vi "BIAS.vi"() -> ()   [LabVIEW 2010]
uses:
  <userlib>/bias/subvis/ROI_rect.ctl
  <userlib>/bias/subvis/Imaging_State.ctl
  <userlib>/bias/subvis/Frame_Controls.ctl
  <vilib>/Utility/error.llb/DialogType.ctl
  <userlib>/bias/classes/CameraBase/CameraBase.lvclass
  <vilib>/event_ctls.llb/lveventtype.ctl
  <userlib>/bias/subvis/zlock/ZLock.lvclass
  <userlib>/bias/subvis/ExposureSettings.ctl
  <vilib>/addons/h5labview2/file/H5Fmode.ctl
  <vilib>/addons/h5labview2/base/hid_t.ctl
  <vilib>/addons/h5labview2/attrib/H5Aread.llb/H5Aread.xnode
  <vilib>/addons/h5labview2/dataset/H5Dread.llb/H5Dread.xnode
  <vilib>/addons/h5labview2/attrib/H5Awrite.llb/H5Awrite.xnode
  <vilib>/Utility/file.llb/Read From Spreadsheet File (DBL).vi
  <vilib>/addons/h5labview2/base/lib_path.vi
  <vilib>/addons/h5labview2/base/H5Equery.vi
  <vilib>/Analysis/NI_AALPro.lvlib
  <vilib>/addons/zeromq/zeromq.lvlib
  <vilib>/addons/h5labview2/file/H5F.lvlib
  <vilib>/addons/h5labview2/group/H5G.lvlib
  <vilib>/addons/h5labview2/attrib/H5A.lvlib
panel:
  in  "files":T1 caption="Files"
  in  "stop":bool
  in  "fit_buttons":cluster{"selection":bool, "stored":bool} caption="Fit"
  in  "tools_zoom":T2 caption="Zoom tools"
  in  "tools_view":cluster{"sel":bool, "in":bool, "out":bool} caption="View tools"
  in  "capture":T3 caption="Capture"
  out "stop_time":dbl=11.582550000000003
  out "busy":bool caption="Busy"
  out "recent_error":bool caption="Error"
  out "remote":bool caption="Remote"
  out "acquiring":bool caption="Acquiring"
  out "img_OD":T4(plugin-control)
  out "n_atoms":dbl caption="Atom number:" format="%_4e"
  out "image_raw":sgl[][](array[numeric])
  in  "tabs":T5(tab)
  in  "store_settings":bool
  in  "binning":cluster{"x":u8, "y":u8}={"x"=1, "y"=1}
  in  "newinst":bool
  in  "effective_pixel":dbl caption="effective pixel size"
  in  "rotation":u16(ring) items=["Do not rotate", "Rotate 90°", "Rotate 180°", "Rotate -90°"]
  out "cam_params":cluster{"String":string, "value":variant}[](array[cluster])=[{"String"="TriggerSource", "value"=variant(string "Freerun")}, {"String"="Timeout", "value"=variant(u32 23583)}, {"String"="ShiftPixelBits", "value"=variant(bool FALSE)}, {"String"="PixelFormat", "value"=variant(string "Mono14")}] caption="Camera Parameters"
  in  "rois":T7(array[cluster])=[{"get"=FALSE, "set"=FALSE, "rect"={"left"=0, "top"=0, "right"=0, "bottom"=0}, "color"=16777224}, {"get"=FALSE, "set"=FALSE, "rect"={"left"=0, "top"=0, "right"=0, "bottom"=0}, "color"=6618880}, {"get"=FALSE, "set"=FALSE, "rect"={"left"=0, "top"=0, "right"=0, "bottom"=0}, "color"=16776960}, {"get"=FALSE, "set"=FALSE, "rect"={"left"=0, "top"=0, "right"=0, "bottom"=0}, "color"=4849919}]
  in  "camera name":string
  out "camera model":string="GX1920 (02-2410B), serial 0xF3101FDAB"
  in  "exposure":sgl=100.0 caption="exposure (ms)"
  out "location":string caption="camera location"
  out "roi_sensor":T6={"left"=0, "top"=0, "right"=1936, "bottom"=1456} caption="camera size"
  out "roi_capture":T6={"left"=686, "top"=399, "right"=1281, "bottom"=1004}
  out "keep":u8
  in  "pedestal":u16=100 caption="Camera pedestal value"
  in  "comp_Isat":bool=TRUE caption="compute?"
  in  "Isat":dbl=4300.0
  in  "Icutoff":dbl=500.0 caption="Intensity threshold"
  in  "xsection":dbl=2.9049e-13 caption="Transition Cross-section"
  out "working dir":path
  out "current file":string
  in  "comp_list":i32(listbox) caption="Computed Frames"
  in  "raw_ctrls":T8={"col_scheme"=0, "val_min"=100.0, "val_max"=16384.0, "automax"=FALSE} {"col_scheme" items=["Grayscale", "Rainbow", "Temperature", "-", "AlpineColors", "Amherst", "Aquamarine", "ArmyColors", "AtlanticColors", "AuroraColors", "AvocadoColors", "BeachColors", "BlueGreenYellow", "BrassTones", "BrightBands", "BrownCyanTones", "CandyColors", "CherryTones", "CMYKColors", "CoffeeTones", "DarkBands", "DarkRainbow", "DarkTerrain", "DeepSeaColors", "Default", "FallColors", "FruitPunchColors", "FuchsiaTones", "GrayTones", "GrayYellowTones", "GreenBrownTerrain", "GreenPinkTones", "IslandColors", "LabVIEW", "LakeColors", "LightTemperatureMap", "LightTerrain", "MintColors", "NeonColors", "NIST", "Pastel", "PearlColors", "PigeonTones", "PlumColors", "Rainbow", "RedBlueTones", "RedGreenSplit", "RoseColors", "RustTones", "SandyTerrain", "SiennaTones", "SolarColors", "SouthwestColors", "StarryNightColors", "SunsetColors", "TemperatureMap", "ThermometerColors", "ValentineTones", "WatermelonColors"]; "val_max" format="%_4g"; "val_min" format="%_4g"}
  in  "comp_ctrls":T8={"col_scheme"=39, "val_min"=0.0, "val_max"=3.0, "automax"=FALSE} {"col_scheme" items=["Grayscale", "Rainbow", "Temperature", "-", "AlpineColors", "Amherst", "Aquamarine", "ArmyColors", "AtlanticColors", "AuroraColors", "AvocadoColors", "BeachColors", "BlueGreenYellow", "BrassTones", "BrightBands", "BrownCyanTones", "CandyColors", "CherryTones", "CMYKColors", "CoffeeTones", "DarkBands", "DarkRainbow", "DarkTerrain", "DeepSeaColors", "Default", "FallColors", "FruitPunchColors", "FuchsiaTones", "GrayTones", "GrayYellowTones", "GreenBrownTerrain", "GreenPinkTones", "IslandColors", "LabVIEW", "LakeColors", "LightTemperatureMap", "LightTerrain", "MintColors", "NeonColors", "NIST", "Pastel", "PearlColors", "PigeonTones", "PlumColors", "Rainbow", "RedBlueTones", "RedGreenSplit", "RoseColors", "RustTones", "SandyTerrain", "SiennaTones", "SolarColors", "SouthwestColors", "StarryNightColors", "SunsetColors", "TemperatureMap", "ThermometerColors", "ValentineTones", "WatermelonColors"]; "val_max" format="%_4g"; "val_min" format="%_4g"}
  in  "raw_list":i32(listbox)=-1 caption="Raw Frames"
  in  "alpha":dbl=1.0 caption="Alpha"
  in  "hold_frames":bool caption="Hold last flat/dark frames"
  in  "histograms":bool caption="histogram"
  in  "Save OD":bool=TRUE
  in  "fit_function":enum16{"Gaussian", "ThomasFermi"}(ring)
  in  "fit clip":dbl=5.0 caption="OD clip" min=1.0
  out "fit_current":bool caption="Current"
  out "fit_number":dbl caption="Fitted atom number:"
  in  "bin_size":i32=5 caption="rebin size" min=1
  out "fit_params":T9(array[cluster])=[{"param"="Fit_residuals", "uncert"=0.0, "uncert 2"=0.0}, {"param"="Fit_rebin", "uncert"=0.0, "uncert 2"=0.0}, {"param"="Gaussian_X0", "uncert"=0.12302468141779599, "uncert 2"=0.0}, {"param"="Gaussian_Y0", "uncert"=0.17648801424407168, "uncert 2"=0.0}, {"param"="Gaussian_XW", "uncert"=0.11674772619735485, "uncert 2"=0.0}, {"param"="Gaussian_YW", "uncert"=0.16283739371170114, "uncert 2"=0.0}, {"param"="Gaussian_Amp", "uncert"=0.008479207725537119, "uncert 2"=0.0}, {"param"="Gaussian_Offset", "uncert"=0.003580147540181461, "uncert 2"=0.0}, {"param"="Gaussian_Nint", "uncert"=1132011.7271960815, "uncert 2"=0.0}] caption="Fit Results" {"uncert 2" format="%#_4g"; "uncert" format="%#_4g"}
  in  "auto fit":bool caption="Auto fit"
  out "data points:":u32=7656 caption="Npoints"
  out "Y-lineout":dbl[][](graph)
  out "X-lineout":dbl[][](graph)
  in  "fit_roi":T10={"get"=FALSE, "set"=FALSE, "rect"={"left"=792, "top"=473, "right"=1233, "bottom"=911}, "color"=16711680} caption="Fitting region"
  out "recent":string[](array[string]) caption="recent log messages"
  out "state":T11 caption="system state"
  in  "last error":T12={"status"=FALSE, "code"=42, "description"="", "time"=timestamp(3029490000.67111 s since 1904-01-01)} caption="most recent error:" {"time" format="%<%H:%M:%S %d/%m/%y>T"}
  out "sequencer":T13(array[cluster])
  out "comp_data":T14(array[cluster])
  out "roi_current":T6
  out "image_data":u16[][][](array[numeric])
  out "frame":i32=-1 caption="display_frame"
  out "fit attribs":variant[](array[variant])
  out "BLACS port":u16
  in  "calc timeout":u32=10000
  out "image_size":i32[](array[numeric])
  out "attribs":variant[](array[variant])=[variant(i32 864), variant(i32 519), variant(i32 1176), variant(i32 878), variant(i64 0), variant(string "Freerun"), variant(u32 1), variant(u32 1), variant(i64 864), variant(i64 519), variant(i64 312), variant(i64 359), variant(dbl 100000.00149011612)]
  out "raw histograms":T15(array[cluster])
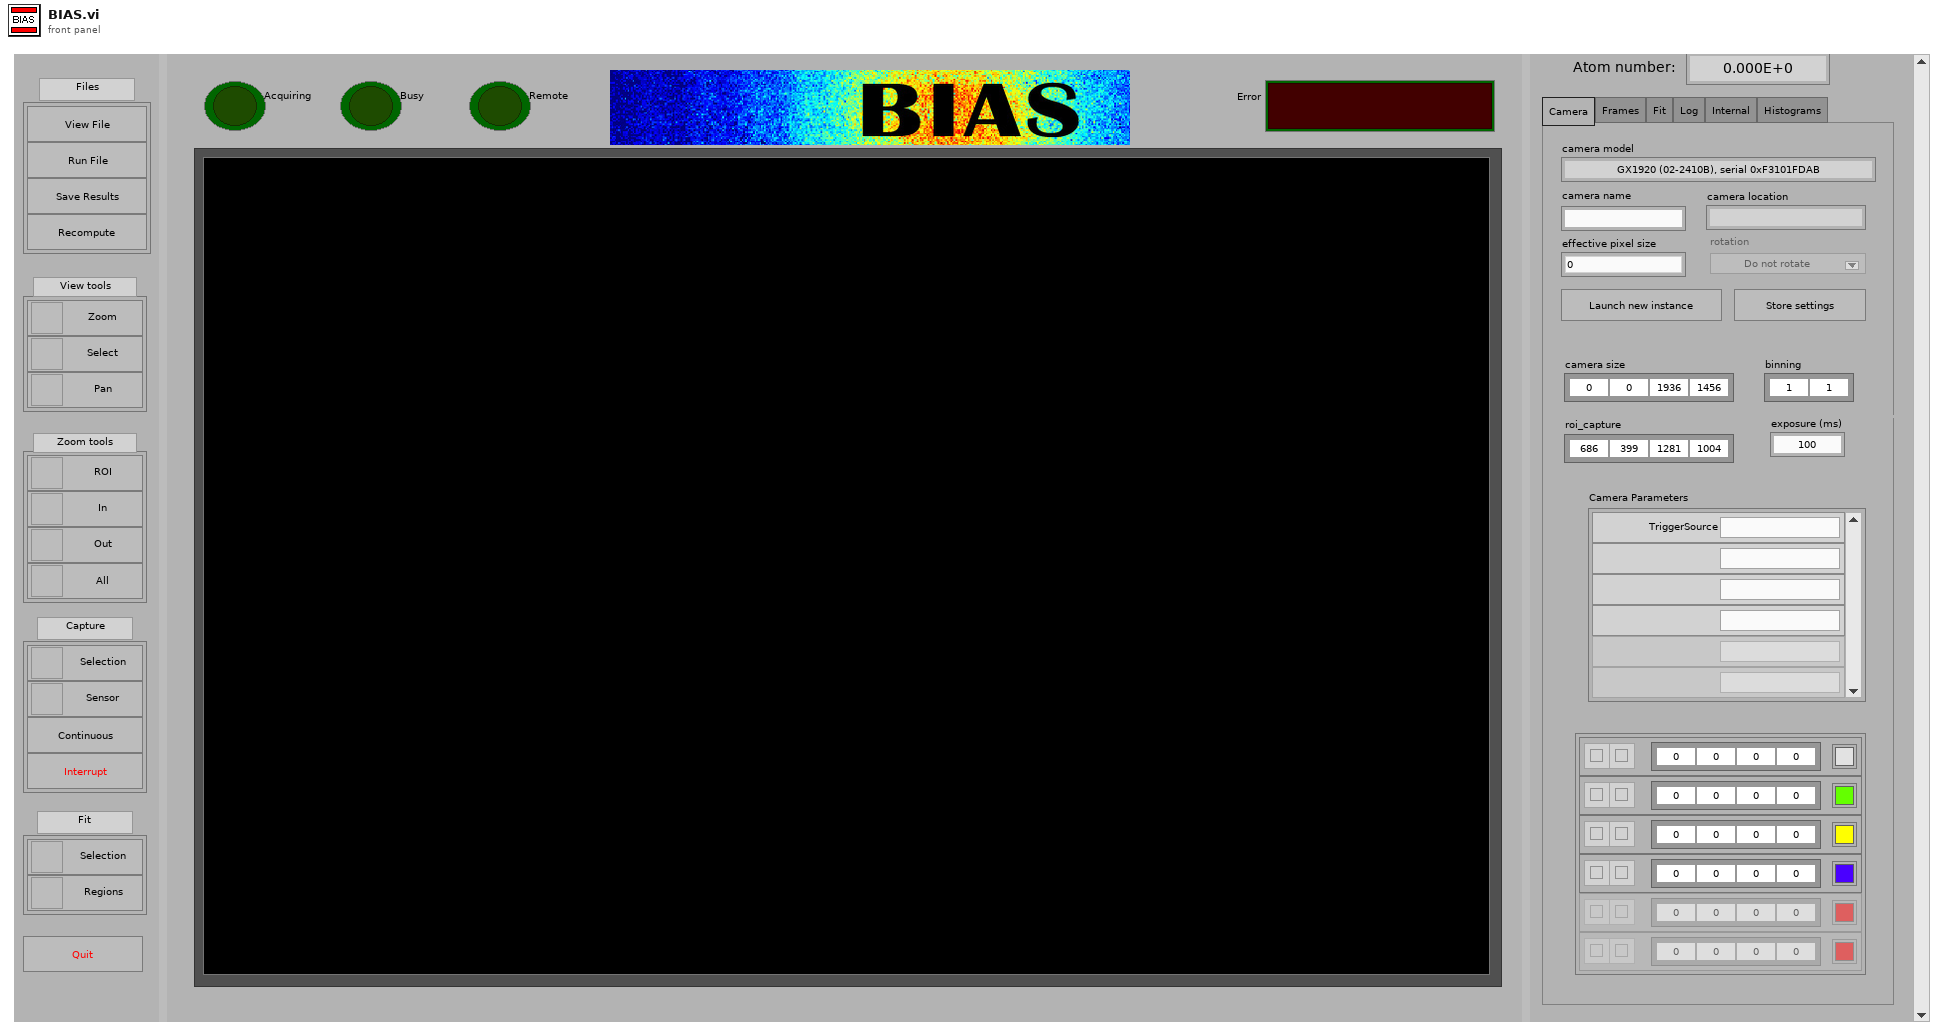
[diagram p1: front panel]
types:
  T1 = cluster{"open_file 2":bool, "open_file":bool, "save_file":bool, "open_file 3":bool}
  T2 = cluster{"sel":bool, "in":bool, "out":bool, "all":bool}
  T3 = cluster{"roi":bool, "chip":bool, "continuous":bool, "abort":bool}
  T4 = typedef "IMAQ Image.ctl" = refnum<image>
  T5 = enum32{"Camera", "Frames", "Fit", "Log", "Internal", "Histograms"}
  T6 = typedef "ROI_rect.ctl" = cluster{"left":i32, "top":i32, "right":i32, "bottom":i32}
  T7 = cluster{"get":bool, "set":bool, "rect":T6, "color":u32}[]
  T8 = typedef "Frame_Controls.ctl" = cluster{"col_scheme":u16, "val_min":sgl, "val_max":sgl, "automax":bool}
  T9 = cluster{"param":string, "uncert":dbl, "uncert 2":dbl}[]
  T10 = cluster{"get":bool, "set":bool, "rect":T6, "color":u32}
  T11 = typedef "Imaging_State.ctl" = enum16{"<NULL>", "Init", "Read File", "Save File", "Idle", "Compute", "Redraw", "Draw Overlays", "Software trigger", "Acquire", "Fit", "Clear", "Quit"}
  T12 = cluster{"status":bool, "code":i32, "description":string, "time":timestamp}
  T13 = cluster{"name":string, "shots":string[], "ids":i32[]}[]
  T14 = cluster{"sequence":string, "name":string, "data":sgl[][], "params":variant[]}[]
  T15 = cluster{"XY Graph":cluster{"X Values":dbl[], "Histogram: h(x)":i32[]}}[]
  T16 = typedef "DialogType.ctl" = u16
  T17 = typedef "pointer.ctl" = u64
  T18 = typedef "ExposureSettings.ctl" = cluster{"exposure":dbl, "external":bool, "roi":T6, "frames":i32, "binning":cluster{"x":u8, "y":u8}}
  T19 = cluster{"Icutoff":dbl, "Isat":dbl, "sigma":dbl, "pixel_size":dbl}
  T20 = typedef "H5F.lvlib/H5Fmode.ctl" = enum16{"read-only", "read-write", "overwrite", "create new", "open or create"}
  T21 = enum8{"Enabled", "Disabled", "Disabled and Grayed Out"}
  T22 = typedef "Image Type" = u32
  T23 = cluster{"sensor_width":u16, "sensor_width":u16, "sensor_width":u16, "sensor_height":u16}
  T24 = cluster{"sequence":string, "name":string, "data":sgl[][], "params":variant[]}
  T25 = cluster{"X Values":dbl[], "Histogram: h(x)":i32[]}
  T26 = cluster{"Histogram Graph":cluster{"X Values":dbl[], "Histogram: h(x)":i32[]}}
  T27 = typedef "hid_t.ctl" = i32
  T28 = cluster{"name":string, "shots":string[], i32[]}[]
  T29 = cluster{"Name":string, "Name":string, "data":sgl[][], "params":variant[]}[]
  T30 = enum32{"Invalid", "Standard", "Closed", "Hidden", "Minimized", "Maximized"}
  T31 = typedef "lveventtype.ctl" = enum32{"Null", "Timeout", "App Instance Close", "App Instance Close?", "Autoscale Range Change", "Cell Edit", "Cell Edit?", "Cursor Grab", "Cursor Grab?", "Cursor Move", "Cursor Release", "Data Change", "Direction Change", "Display State Change", "Drag Ended", "Drag Enter", "Drag Leave", "Drag Over", "Drag Source Update", "Drag Starting", "Drag Starting?", "Drop", "Exec State Change", "Key Down", "Key Down?", "Key Repeat", "Key Repeat?", "Key Up", "Listbox Double Click", "Menu Activation?", "Menu Selection (App)", "Menu Selection? (App)", "Menu Selection (User)", "Mouse Down", "Mouse Down?", "Mouse Enter", "Mouse Leave", "Mouse Move", "Mouse Up", "NI Security User Change (App)", "Pane Size", "Panel Close", "Panel Close?", "Panel Resize", "Plot Attribute Change", "Scale Range Change", "Shortcut Menu Activation?", "Shortcut Menu Selection (App)", "Shortcut Menu Selection? (App)", "Shortcut Menu Selection (User)", "Tree Double Click", "Tree Drag", "Tree Drag?", "Tree Drop", "Tree Drop?", "Tree Item Close", "Tree Item Close?", "Tree Item Open", "Tree Item Open?", "Value Change"}
  T32 = cluster{"Global Rectangle":i32[], "Contours":cluster{"Contour Type":u32, "ROI Type":u32, "Points":i32[]}[]}
  T33 = typedef "ROI Descriptor" = cluster{"Global Rectangle":i32[], "Contours":cluster{"ID":enum32{"External", "Internal"}, "Type":u32, "Coordinates":i32[]}[]}
  T34 = cluster{"Contour Type":u32, "ROI Type":u32, "Points":i32[]}[]
  T35 = cluster{"FinalVal[0]":bool, "FinalVal[1]":bool, "FinalVal[2]":bool}
  T36 = cluster{"all rows[0]":dbl, "all rows[1]":dbl, "all rows[2]":dbl}
  T37 = cluster{"Value":u8, "Value":u8, "Value":u8, "Value":u8}
  T38 = enum16{"Standard", "Buffered", "CRLF", "Immediate"}
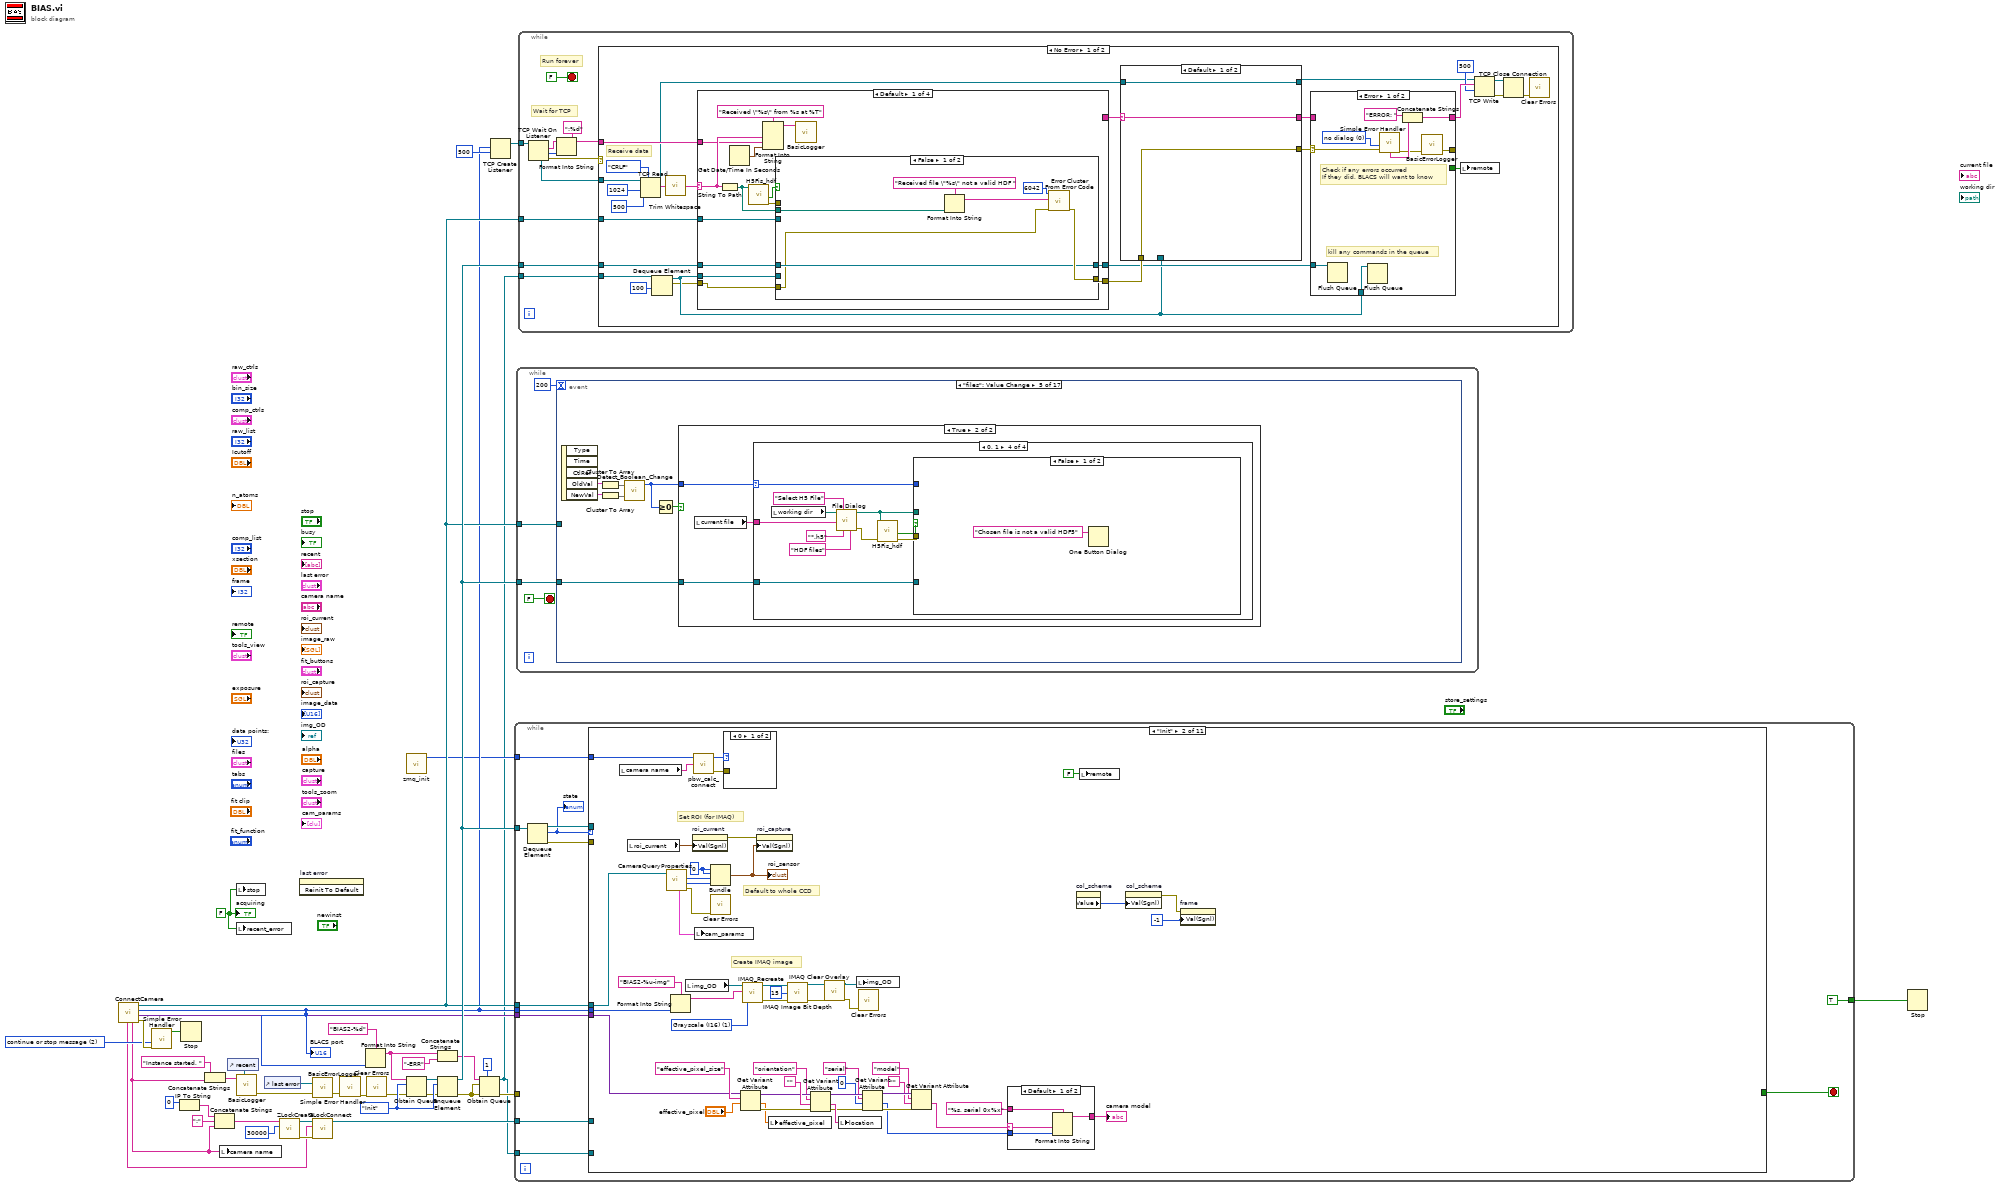
[diagram p0: block diagram]
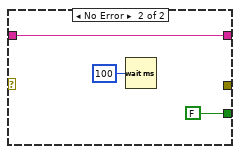
[diagram p2: hidden frame]
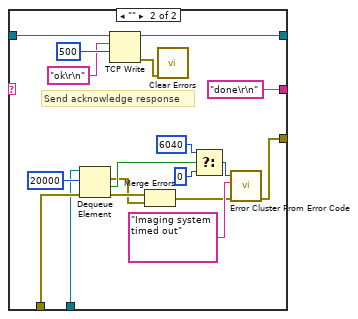
[diagram p3: hidden frame]
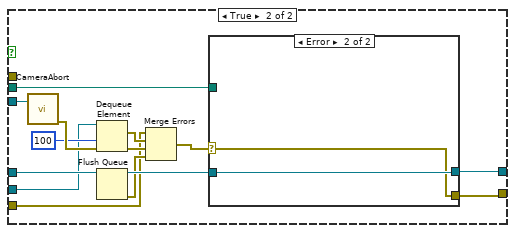
[diagram p4: hidden frame]
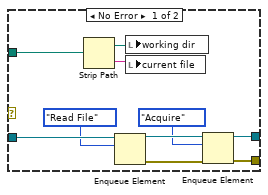
[diagram p5: hidden frame]
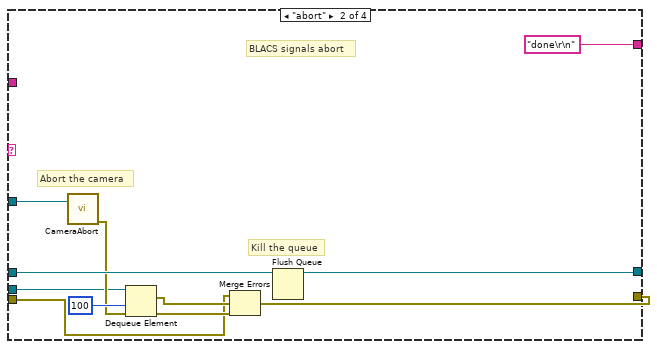
[diagram p6: hidden frame]
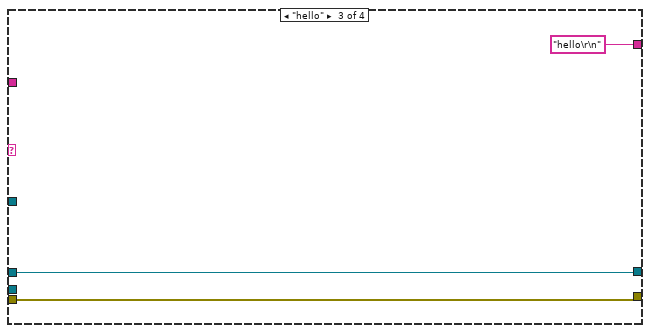
[diagram p7: hidden frame]
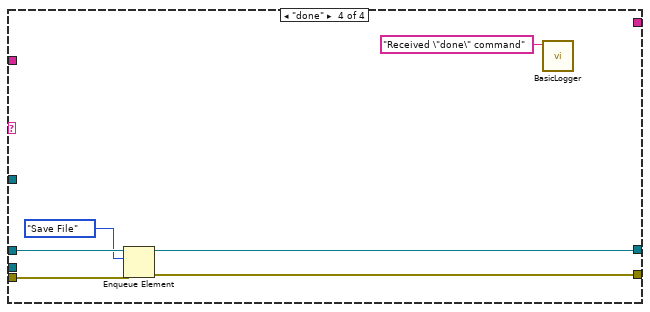
[diagram p8: hidden frame]
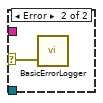
[diagram p9: hidden frame]
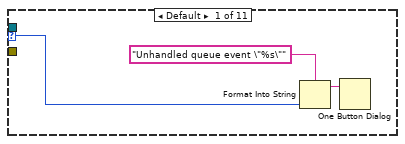
[diagram p10: hidden frame]
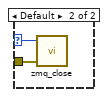
[diagram p11: hidden frame]
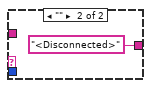
[diagram p12: hidden frame]
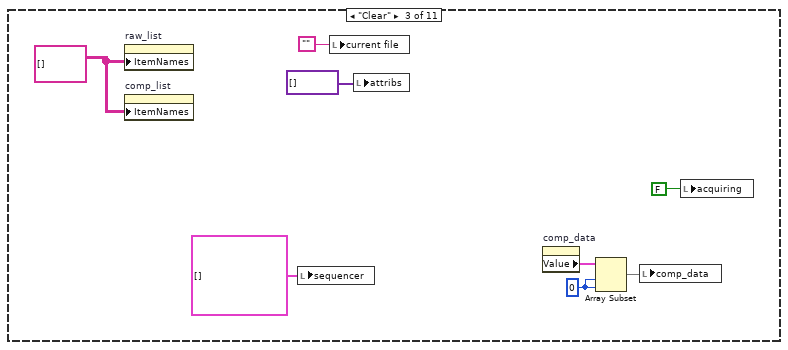
[diagram p13: hidden frame]
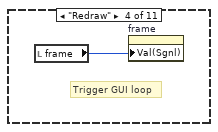
[diagram p14: hidden frame]
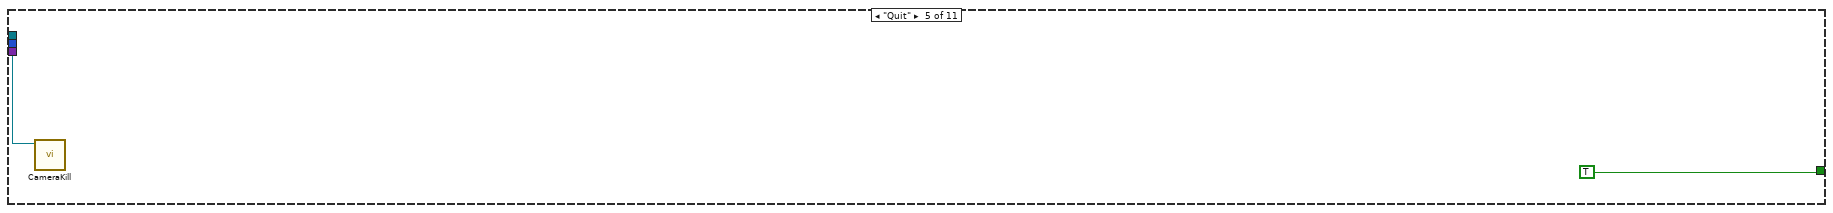
[diagram p15: hidden frame]
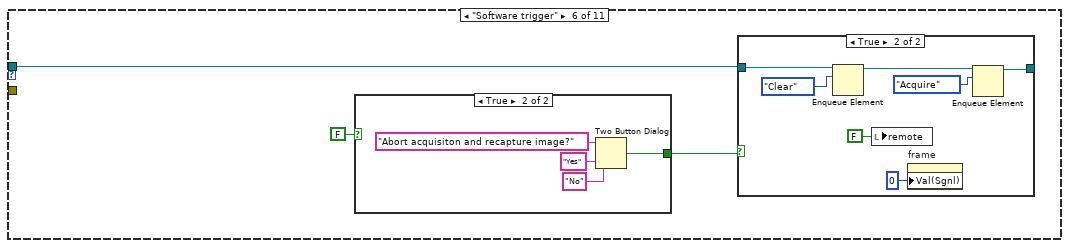
[diagram p16: hidden frame]
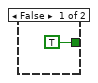
[diagram p18: hidden frame]
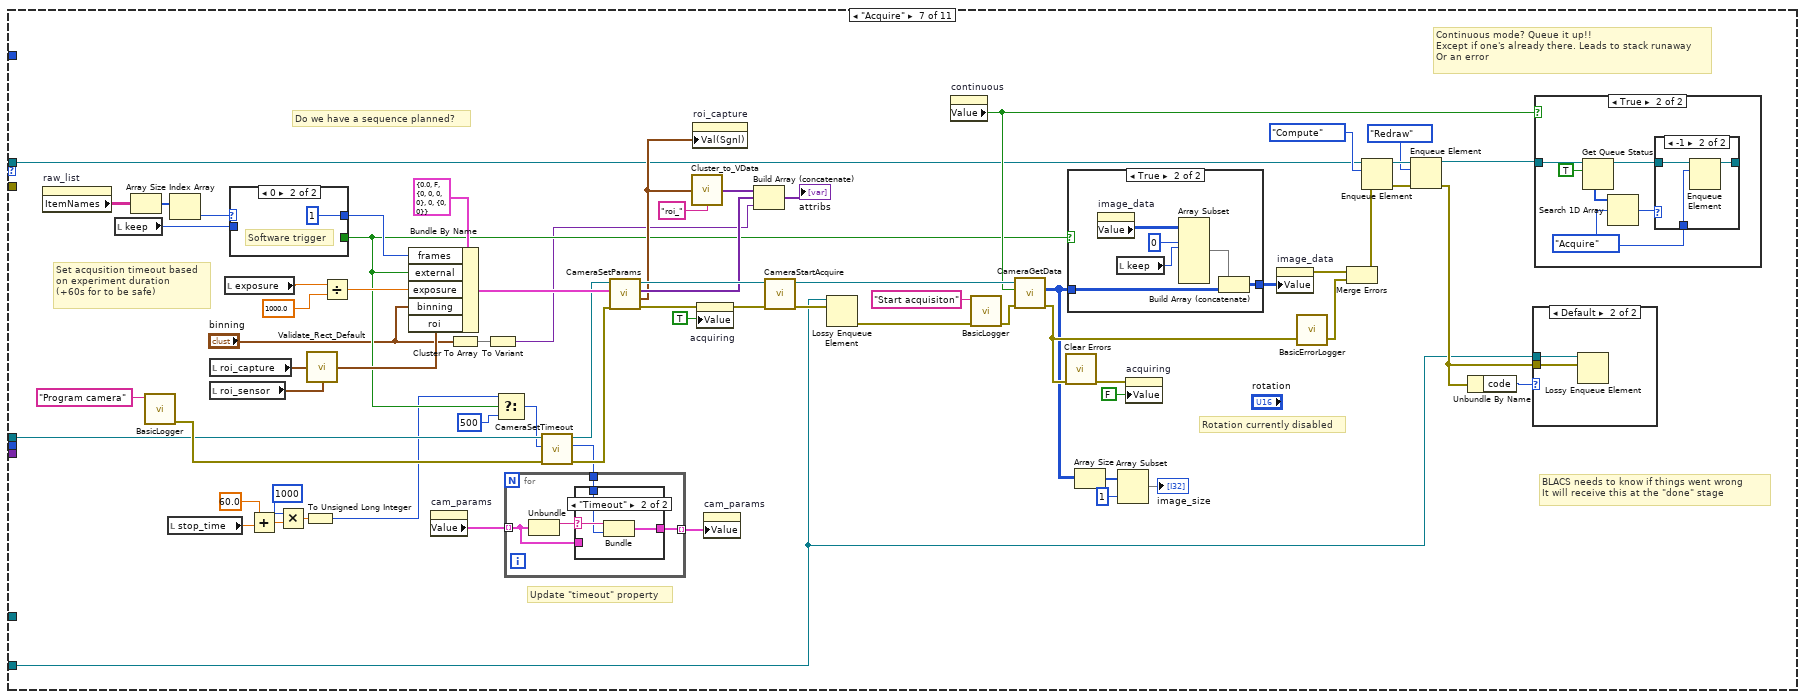
[diagram p19: hidden frame]
diagram:
  w20 = T16 2 items=["no dialog", "OK message", "continue or stop message", "OK message + warnings", "continue/stop + warnings"] ("type of dialog (OK msg:1)")
  w26 = FALSE ("acquiring")
  w40 = Imaging_State."Init" ("Imaging_State")
  n1 = call <userlib>:"ConnectCamera.vi"() -> ("error out"=w22:errorcluster, "params"=w10:variant, "port"=w23:u16, "camera"=w24:refnum<class "CameraBase.lvclass">, "camera name"=w9:string, "zlock"=w11:string)  [unwired: 3 in, 1 out]
  "BLACS port" <- w23
  n2 = call <vilib>:"Simple Error Handler.vi"("type of dialog (OK msg:1)"=w20, "error in (no error)"=w22) -> ("error?"=w21:bool)  [unwired: 3 in, 4 out]
  n3 = IP To String(2:u32 0 ("net address")) -> (0:w15:string)  [unwired: 1 in]
  n4 = Stop(stop? (T)=w21) -> ()
  n5 = Concatenate Strings("Instance started, " ("string"), w9) -> (w27:string)
  n6 = Concatenate Strings(w15, ":" ("string"), w9) -> (w16:string)
  n7 = local write "camera name"(w9) -> ()
  n8 = control-ref of="recent"() -> (w29:refnum<vi>)
  n9 = local write "stop"(w26) -> ()
  n10 = local write "recent_error"(w26) -> ()
  n11 = call <userlib>:"BasicLogger.vi"("indicator"=w29, "text"=w27) -> ("error out"=w30:errorcluster)  [unwired: 5 in, 1 out]
  n12 = control-ref of="last error"() -> (w34:refnum<vi>)
  n13 = call <userlib>:"ZLockCreate.vi"("timeout (500ms)"=30000, "app name"=w16) -> ("error out"=w18:errorcluster, "ZLock out"=w19:refnum<class "ZLock.lvclass">)  [unwired: 4 in]
  n14 = invoke on="last error" class="Clust (strict)" method="Reinit To Default"() -> ()  [unwired: 3 in, 3 out]
  n15 = call <userlib>:"BasicErrorLogger.vi"("error in"=w30, "indicator"=w34) -> ("error out"=w33:errorcluster)  [unwired: 1 out]
  n16 = call-dynamic "ZLockConnect.vi"("error in (no error)"=w18, "host"=w11, "ZLock in"=w19) -> ("ZLock out"=w17:refnum<class "ZLock.lvclass">)  [unwired: 7 in, 1 out]
  n17 = call <vilib>:"Simple Error Handler.vi"("error in (no error)"=w33) -> ("error out"=w32:errorcluster)  [unwired: 4 in, 4 out]
  n18 = Format Into String(format string="BIAS2-%d" ("name (unnamed)"), w23) -> (resulting string=w7:string)  [unwired: 2 in, 1 out]
  n19 = call <vilib>:"Clear Errors.vi"("error in (no error)"=w32) -> ("error out"=w31:errorcluster)  [unwired: 6 in]
  n20 = call <vilib>:"zmq_init.vi"() -> ("context"=w12:T17)  [unwired: 4 in, 1 out]
  n21 = Obtain Queue(name (unnamed)=w7, element data type=w40, error in (no error)=w31) -> (queue out=w41:refnum<queue>, error out=w39:errorcluster)  [unwired: 2 in, 1 out]
  n22 = Concatenate Strings(w7, "-ERR" ("name (unnamed)")) -> (w5:string)
  n23 = Enqueue Element(queue=w41, element=w40, error in (no error)=w39) -> (queue out=w36:refnum<queue>, error out=w4:errorcluster)  [unwired: 1 in, 1 out]
  n24 = Obtain Queue(max queue size (-1, unlimited)=1, name (unnamed)=w5, element data type=w4, error in (no error)=w4) -> (queue out=w1:refnum<queue>, error out=w8:errorcluster)  [unwired: 1 in, 1 out]
  n25 = TCP Create Listener(9:500 ("timeout ms (25000)"), 10:w23) -> (3:w35:refnum<k5>)  [unwired: 3 in, 2 out]
  n26 = while {
    tunnel: [TRUE] -> w38
    tunnel: w24 -> [w49]
    tunnel: w36 -> [w44]
    tunnel: w12 -> [w48]
    tunnel: w17 -> [w47]
    tunnel: w23 -> [w46]
    tunnel: w10 -> [w43]
    tunnel: w8 -> [_]
    tunnel: w1 -> [w42]
    stop <- w50 stop-if-true
    n27 = Dequeue Element(queue=w44) -> (queue out=w53:refnum<queue>, element=w45:T11, error out=w52:errorcluster)  [unwired: 2 in, 1 out]
    "state" <- w45
    n28 = case shown="\"Init\"" w45 {
      selector: w45 -> [w55 _ _ _ _ _ _ _ _ _ _]
      tunnel: w53 -> [_ _ _ _ _ w126 w145 w251 _ w439 w673]
      tunnel: w52 -> [_ _ _ _ _ _ _ _ _ _ _]
      tunnel: [_ _ _ _ TRUE _ _ _ _ _ _] -> w50
      tunnel: w49 -> [_ w89 _ _ w123 _ w179 _ _ _ _]
      tunnel: w48 -> [_ w82 _ _ _ _ _ w245 w346 _ _]
      tunnel: w47 -> [_ _ _ _ _ _ _ _ _ w434 w674]
      tunnel: w46 -> [_ w79 _ _ _ _ _ _ _ _ _]
      tunnel: w43 -> [_ w63 _ _ _ _ _ _ _ _ _]
      tunnel: w42 -> [_ _ _ _ _ _ w141 _ _ w433 w672]
      frame Default {
        n29 = Format Into String(format string="Unhandled queue event \"%s\"", w55) -> (resulting string=w54:string)  [unwired: 2 in, 1 out]
        n30 = One Button Dialog(message=w54) -> ()  [unwired: 1 in, 1 out]
      }
      frame "Init" {
        w88 = u16 0 ("sensor_width")
        w105 = T22 1 items=["Grayscale (U8)", "Grayscale (I16)", "Grayscale (SGL)", "Complex (CSG)", "RGB (U32)", "HSL (U32)", "RGB (U64)", "Grayscale (U16)"] ("type")
        # "Create IMAQ image"
        # "Default to whole CCD"
        # "Set ROI (for IMAQ)"
        n31 = local read "camera name"() -> (w80:string)
        n32 = local read "roi_current"() -> (w100:T6)
        n33 = call-dynamic "CameraQueryProperties.vi"("CameraBase in"=w89) -> ("error out"=w90:errorcluster, "sensor_height"=w99:u16, "sensor_width"=w98:u16, "cam_params"=w97:cluster{"String":string, "value":variant}[])  [unwired: 6 in, 1 out]
        n34 = Format Into String(format string="BIAS2-%u-img", w79) -> (resulting string=w83:string)  [unwired: 2 in, 1 out]
        n35 = local read "img_OD"() -> (w106:T4)
        n36 = property on="roi_current" class="Clust (strict)"("Val(Sgnl)"=w100) -> (error out=w101:errorcluster)  [unwired: 2 in, 1 out]
        n37 = call <userlib>:"pbw_calc_connect.vi"("identity"=w80, "ctx in"=w82) -> ("error out"=w81:errorcluster, "socket out"=w57:T17)  [unwired: 2 in]
        n38 = local write "cam_params"(w97) -> ()
        n39 = Bundle("sensor_width"=w88, "sensor_width"=w88, "sensor_width"=w98, "sensor_height"=w99) -> (w85:T23)  [unwired: 1 in]
        "roi_sensor" <- w85
        n40 = call <vilib>:"Clear Errors.vi"("error in (no error)"=w90) -> ()  [unwired: 6 in, 1 out]
        n41 = case shown="0" w57 {
          selector: w57 -> [_ w107]
          tunnel: w81 -> [_ w108]
          frame 0 {
          }
          frame Default {
            n42 = call <vilib>:"zmq_close.vi"("error in"=w108, "socket in"=w107) -> ()  [unwired: 3 in, 1 out]
          }
        }
        n43 = Get Variant Attribute(Variant=w63, name="effective_pixel_size", default value (empty Variant)="effective_pixel") -> (duplicate Variant=w72:variant, value=w65:dbl, error out=w75:errorcluster)  [unwired: 1 in, 1 out]
        n44 = call <userlib>:"IMAQ_Recreate.vi"("type"=w105, "name"=w83, "image in"=w106) -> ("error out"=w102:errorcluster, "image out"=w104:T4)  [unwired: 3 in]
        n45 = property on="roi_capture" class="Clust (strict)"(error in=w101, "Val(Sgnl)"=w85) -> ()  [unwired: 1 in, 2 out]
        n46 = local write "effective_pixel"(w65) -> ()
        n47 = call "IMAQ Image Bit Depth"("Image"=w104, "Bit Depth (0)"=u32 15, "error in (no error)"=w102) -> ("Image Out"=w95:T4, "error out"=w96:errorcluster)  [unwired: 10 in, 1 out]
        n48 = Get Variant Attribute(Variant=w72, name="orientation", default value (empty Variant)="", error in=w75) -> (duplicate Variant=w73:variant, value=w77:string, error out=w76:errorcluster)  [unwired: 1 out]
        n49 = call "IMAQ Clear Overlay"("error in (no error)"=w96, "Image"=w95) -> ("error out"=w93:errorcluster, "Image Out"=w94:T4)  [unwired: 8 in]
        n50 = local write "location"(w77) -> ()
        n51 = local write "img_OD"(w94) -> ()
        n52 = call <vilib>:"Clear Errors.vi"("error in (no error)"=w93) -> ()  [unwired: 6 in, 1 out]
        n53 = Get Variant Attribute(Variant=w73, name="serial", default value (empty Variant)=u64 0, error in=w76) -> (duplicate Variant=w70:variant, value=w68:u64, error out=w71:errorcluster)  [unwired: 1 out]
        n54 = Get Variant Attribute(Variant=w70, name="model", default value (empty Variant)="", error in=w71) -> (value=w69:string)  [unwired: 3 out]
        n55 = case shown="Default" w69 {
          selector: w69 -> [w110 _]
          tunnel: [w112 "<Disconnected>"] -> w59
          tunnel: w68 -> [w111 _]
          tunnel: "%s, serial 0x%x" ("format string") -> [w109 _]
          frame Default {
            n56 = Format Into String(format string=w109, w110, w111) -> (resulting string=w112:string)  [unwired: 2 in, 1 out]
          }
          frame "" {
          }
        }
        "camera model" <- w59
        n57 = property on="col_scheme" class="Ring (strict)"() -> ("Value"=w91:u16)  [unwired: 2 in, 2 out]
        n58 = local write "remote"(FALSE ("remote")) -> ()
        n59 = property on="col_scheme" class="Ring (strict)"("Val(Sgnl)"=w91) -> (error out=w86:errorcluster)  [unwired: 2 in, 1 out]
        n60 = property on="frame" class="DigNum (strict)"(error in=w86, "Val(Sgnl)"=-1 ("display_frame")) -> ()  [unwired: 1 in, 2 out]
      }
      frame "Clear" {
        w116 = 0 ("index")
        w119 = string[][] [] ("sequence")
        n61 = property on="raw_list" class="MCListbox (strict)"("ItemNames"=w119) -> ()  [unwired: 2 in, 2 out]
        n62 = property on="comp_list" class="MCListbox (strict)"("ItemNames"=w119) -> ()  [unwired: 2 in, 2 out]
        n63 = local write "sequencer"(T13 [] ("sequencer")) -> ()
        n64 = local write "current file"("") -> ()
        n65 = local write "attribs"(variant[] []) -> ()
        n66 = property on="comp_data" class="Arr (strict)"() -> ("Value"=w114:T14)  [unwired: 2 in, 2 out]
        n67 = Array Subset(array=w114, index=w116, length=w116) -> (w117:T14)
        n68 = local write "comp_data"(w117) -> ()
        n69 = local write "acquiring"(FALSE ("pending")) -> ()
      }
      frame "Redraw" {
        # "Trigger GUI loop"
        n70 = local read "frame"() -> (w122:i32)
        n71 = property on="frame" class="DigNum (strict)"("Val(Sgnl)"=w122) -> ()  [unwired: 2 in, 2 out]
      }
      frame "Quit" {
        n72 = call-dynamic "CameraKill.vi"("CameraBase in"=w123) -> ()  [unwired: 9 in, 2 out]
      }
      frame "Software trigger" {
        n73 = case shown="True" FALSE {
          tunnel: [TRUE ("T button?") w137] -> w127
          frame False {
          }
          frame True {
            n74 = Two Button Dialog(message="Abort acquisiton and recapture image?", 1:"No" ("F button name (\"Cancel\")"), 2:"Yes" ("T button name (\"OK\")")) -> (T button?=w137:bool)
          }
        }
        n75 = case shown="True" w127 {
          tunnel: [w128 w134] -> _
          tunnel: w126 -> [w128 w133]
          frame False {
          }
          frame True {
            n76 = Enqueue Element(queue=w133, element=Imaging_State."Clear") -> (queue out=w132:refnum<queue>)  [unwired: 2 in, 2 out]
            n77 = local write "remote"(FALSE ("remote")) -> ()
            n78 = property on="frame" class="DigNum (strict)"("Val(Sgnl)"=0 ("Value (Signaling)")) -> ()  [unwired: 2 in, 2 out]
            n79 = Enqueue Element(queue=w132, element=Imaging_State."Acquire") -> (queue out=w134:refnum<queue>)  [unwired: 2 in, 2 out]
          }
        }
      }
      frame "Acquire" {
        # "Update \"timeout\" property"
        # "Rotation currently disabled"
        # "Set acqusition timeout based\non experiment duration\n(+60s for to be safe)"
        # "BLACS needs to know if things went wrong\nIt will receive this at the \"done\" stage"
        # "Continuous mode? Queue it up!!\nExcept if one's already there. Leads to stack runaway\nOr an error"
        # "Do we have a sequence planned?"
        n80 = property on="raw_list" class="MCListbox (strict)"() -> ("ItemNames"=w190:string[][])  [unwired: 2 in, 2 out]
        n81 = local read "keep"() -> (w183:u8)
        n82 = Array Size(array=w190) -> (size(s)=w189:i32[])
        n83 = call <userlib>:"BasicLogger.vi"("text"="Program camera") -> ("error out"=w180:errorcluster)  [unwired: 6 in, 1 out]
        n84 = local read "stop_time"() -> (w174:dbl)
        n85 = Index Array(array=w189) -> (element=w188:i32)  [unwired: 1 in]
        n86 = local read "roi_capture"() -> (w204:T6)
        n87 = local read "roi_sensor"() -> (w199:T6)
        n88 = local read "exposure"() -> (w208:sgl)
        n89 = case shown="0" w188 {
          selector: w188 -> [w237 _]
          tunnel: [w238 1] -> w165
          tunnel: [TRUE ("external") _] -> w156
          tunnel: w183 -> [w236 _]
          frame Default {
            n90 = Subtract(x=w237, y=w236) -> (x-y=w238:i32)
          }
          frame 0 {
            # "Software trigger"
          }
        }
        n91 = Add(x=60.0, y=w174) -> (x+y=w175:dbl)
        n92 = Multiply(x=u32 1000 ("col"), y=w175) -> (x*y=w182:dbl)
        n93 = To Unsigned Long Integer(number=w182) -> (unsigned 32bit integer=w155:u32)
        n94 = call <userlib>:"Validate_Rect_Default.vi"("rect"=w204, "default"=w199) -> ("out"=w169:T6)
        n95 = Divide(x=w208, y=sgl 1000.0) -> (x/y=w203:sgl)
        n96 = Bundle By Name(cluster=T18 {"exposure"=0.0, "external"=FALSE, "roi"={"left"=0, "top"=0, "right"=0, "bottom"=0}, "frames"=0, "binning"={"x"=0, "y"=0}} ("settings"), "frames"=w165, "external"=w156, "exposure"=w203, "binning"="binning", "roi"=w169) -> (w202:T18)
        n97 = property on="cam_params" class="Arr (strict)"() -> ("Value"=w164:cluster{"String":string, "value":variant}[])  [unwired: 2 in, 2 out]
        n98 = Cluster To Array(cluster="binning") -> (array=w146:u8[])
        n99 = To Variant(anything=w146) -> (Variant=w147:variant)
        n100 = Select(t=w155, s=w156, f=u32 500) -> (s? t:f=w154:u32)
        n101 = call-dynamic "CameraSetTimeout.vi"("error in (no error)"=w180, "Timeout"=w154, "CameraBase in"=w179) -> ("error out"=w178:errorcluster, "Timeout set"=w176:u32, "CameraBase out"=w177:refnum<class "CameraBase.lvclass">)  [unwired: 6 in]
        n102 = for {
          tunnel: w164 -> [w216] mode=indexing
          tunnel: w176 -> [w217]
          tunnel: [w219] -> w163 mode=indexing
          n103 = Unbundle(w216) -> ("String"=w218:string)  [unwired: 1 out]
          n104 = case shown="\"Timeout\"" w218 {
            selector: w218 -> [_ w222]
            tunnel: [w220 w223] -> w219
            tunnel: w217 -> [_ w221]
            tunnel: w216 -> [w220 _]
            frame Default {
            }
            frame "Timeout" {
              n105 = Bundle(w222, "Timeout set"=w221) -> (w223:cluster{string, "Timeout set":u32})  [unwired: 1 in]
            }
          }
        }
        n106 = call-dynamic "CameraSetParams.vi"("error in (no error)"=w178, "settings"=w202, "CameraBase in"=w177) -> ("error out"=w195:errorcluster, "roi_out"=w171:T6, "attributes"=w187:variant[], "CameraBase out"=w194:refnum<class "CameraBase.lvclass">)  [unwired: 5 in]
        n107 = call <userlib>:"Cluster_to_VData.vi"("cluster"=w171, "prefix"="roi_") -> ("vdata"=w186:variant[])
        n108 = property on="roi_capture" class="Clust (strict)"("Val(Sgnl)"=w171) -> ()  [unwired: 2 in, 2 out]
        n109 = property on="acquiring" class="Bool (strict)"(error in=w195, "Value"=TRUE ("acquiring")) -> (error out=w192:errorcluster)  [unwired: 1 in, 1 out]
        n110 = property on="cam_params" class="Arr (strict)"("Value"=w163) -> ()  [unwired: 2 in, 2 out]
        n111 = Build Array (concatenate)(w186, w187, w147) -> (→"attribs":variant[])
        n112 = call-dynamic "CameraStartAcquire.vi"("error in (no error)"=w192, "CameraBase in"=w194) -> ("error out"=w143:errorcluster, "CameraBase out"=w193:refnum<class "CameraBase.lvclass">)  [unwired: 8 in]
        n113 = Lossy Enqueue Element(queue=w141, element=w143) -> (error out=w144:errorcluster)  [unwired: 1 in, 3 out]
        n114 = property on="continuous" class="Bool (strict)"() -> ("Value"=w168:bool)  [unwired: 2 in, 2 out]
        n115 = call <userlib>:"BasicLogger.vi"("error in"=w144, "text"="Start acquisiton") -> ("error out"=w191:errorcluster)  [unwired: 5 in, 1 out]
        n116 = call-dynamic "CameraGetData.vi"("error in (no error)"=w191, "keep open?"=w168, "CameraBase in"=w193) -> ("error out"=w206:errorcluster, "image_data"=w152:u16[][][])  [unwired: 6 in, 1 out]
        n117 = call <vilib>:"Clear Errors.vi"("error in (no error)"=w206) -> ("error out"=w196:errorcluster)  [unwired: 6 in]
        n118 = case shown="True" w156 {
          tunnel: [w209 w212] -> w172
          tunnel: w152 -> [w209 w210]
          frame False {
          }
          frame True {
            n119 = property on="image_data" class="Arr (strict)"() -> ("Value"=w211:u16[][][])  [unwired: 2 in, 2 out]
            n120 = local read "keep"() -> (w214:u8)
            n121 = Array Subset(array=w211, index (dim 0)=0 ("index"), length (dim 0)=w214) -> (w213:u16[][][])  [unwired: 4 in]
            n122 = Build Array (concatenate)(w213, w210) -> (w212:u16[][][])
          }
        }
        n123 = Array Size(array=w152) -> (size(s)=w151:i32[])
        n124 = Array Subset(array=w151, index=1) -> (→"image_size":i32[])  [unwired: 1 in]
        n125 = property on="acquiring" class="Bool (strict)"(error in=w196, "Value"=FALSE ("acquiring")) -> ()  [unwired: 1 in, 2 out]
        n126 = property on="image_data" class="Arr (strict)"("Value"=w172) -> (error out=w167:errorcluster)  [unwired: 2 in, 1 out]
        n127 = call <userlib>:"BasicErrorLogger.vi"("error in"=w206) -> ("error out"=w166:errorcluster)  [unwired: 1 in, 1 out]
        n128 = Merge Errors(w167, w166) -> (w159:errorcluster)
        n129 = Enqueue Element(queue=w145, element=Imaging_State."Compute", error in (no error)=w159) -> (queue out=w162:refnum<queue>, error out=w158:errorcluster)  [unwired: 1 in, 1 out]
        n130 = Enqueue Element(queue=w162, element=Imaging_State."Redraw", error in (no error)=w158) -> (queue out=w142:refnum<queue>, error out=w157:errorcluster)  [unwired: 1 in, 1 out]
        n131 = Unbundle By Name(w157) -> ("code"=w184:i32)
        n132 = case shown="Default" w184 {
          tunnel: w157 -> [_ w225]
          tunnel: w141 -> [_ w224]
          frame 0, 5024 {
            # "Fine or Abort"
          }
          frame Default {
            n133 = Lossy Enqueue Element(queue=w224, element=w225) -> ()  [unwired: 1 in, 4 out]
          }
        }
        n134 = case shown="True" w168 {
          tunnel: w142 -> [_ w231]
          frame False {
          }
          frame True {
            w226 = Imaging_State."Acquire" ("element")
            n135 = Get Queue Status(queue=w231, return elements? (F)=TRUE) -> (queue out=w227:refnum<queue>, elements=w229:T11[])  [unwired: 1 in, 6 out]
            n136 = Search 1D Array(1D array=w229, element=w226) -> (index of element=w228:i32)  [unwired: 1 in]
            n137 = case shown="-1" w228 {
              tunnel: [w232 w235] -> _
              tunnel: w227 -> [w232 w234]
              tunnel: w226 -> [_ w233]
              frame Default {
              }
              frame -1 {
                n138 = Enqueue Element(queue=w234, element=w233) -> (queue out=w235:refnum<queue>)  [unwired: 2 in, 2 out]
              }
            }
          }
        }
      }
      frame "Compute" {
        # ">> num frames >>"
        # "Ensure the fit happens before saving if auto fit enabled."
        n139 = property on="comp_data" class="Arr (strict)" props=["Value"]() -> ()  [unwired: 2 in, 3 out]
        n140 = property on="sequencer" class="Arr (strict)"() -> ("Value"=w246:T13)  [unwired: 2 in, 2 out]
        n141 = property on="raw_list" class="MCListbox (strict)"() -> ("ItemNames"=w254:string[][])  [unwired: 2 in, 2 out]
        n142 = local read "camera name"() -> (w241:string)
        n143 = for {
          N -> [w281]
          tunnel: w246 -> [w285] mode=indexing
          tunnel: [w291] -> w249
          tunnel: w254 -> [w288]
          tunnel: [errorcluster {"status"=FALSE, "code"=0, "source"=""} ("error in (no error)")] -> w250
          tunnel: [w281] -> w252
          tunnel: w245 -> [w280]
          shift-right: [w278] -> w243
          shift-left: T14 [] -> [w279]
          tunnel: w241 -> [w277]
          # ">> sequence >>"
          # "Try to find frames"
          n144 = Unbundle(w285) -> ("name"=w292:string)  [unwired: 2 out]
          n145 = call <userlib>:"Keep_Find.vi"("x"="atoms" ("name"), "sequence"=w285) -> ("index"=w283:i32)  [unwired: 1 in]
          n146 = call <userlib>:"Keep_Find.vi"("x"="flat" ("name"), "rawlist"=w288, "sequence"=w285) -> ("index"=w287:i32)
          n147 = call <userlib>:"Keep_Find.vi"("x"="dark" ("name"), "rawlist"=w288, "sequence"=w285) -> ("index"=w286:i32)
          n148 = Greater Or Equal To 0?(x=w283) -> (x >= 0?=w295:bool)
          n149 = Greater Or Equal To 0?(x=w287) -> (x >= 0?=w294:bool)
          n150 = Compound Arithmetic op=AND(w295, w294) -> (w293:bool)
          n151 = case shown="True" w293 {
            tunnel: w283 -> [_ w334]
            tunnel: w287 -> [_ w332]
            tunnel: w286 -> [_ w333]
            tunnel: w292 -> [_ w331]
            tunnel: [_ w321] -> w291
            tunnel: w280 -> [_ w303]
            tunnel: w279 -> [w296 w298]
            tunnel: [w296 w299] -> w278
            tunnel: w277 -> [_ w297]
            frame False {
            }
            frame True {
              w310 = 1 ("dimension size")
              n152 = property on="image_data" class="Arr (strict)"() -> ("Value"=w314:u16[][][])  [unwired: 2 in, 2 out]
              n153 = local read "effective_pixel"() -> (w301:dbl)
              n154 = Index Array(array=w314, index (dim 0) #1=w334, index (dim 0) #2=w332, index (dim 0) #3=w333) -> (element #1=w304:u16[][], element #2=w305:u16[][], element #3=w307:u16[][])  [unwired: 6 in]
              n155 = local read "xsection"() -> (w318:dbl)
              n156 = Select(t="Isat", s="comp_Isat", f=0.0) -> (s? t:f=w319:dbl)
              n157 = local read "Icutoff"() -> (w320:dbl)
              n158 = Empty Array?(array=w307) -> (empty?=w309:bool)
              n159 = Initialize Array("pedestal", w310, w310) -> (w308:u16[][])
              n160 = Bundle By Name(cluster=T19 {"Icutoff"=0.0, "Isat"=0.0, "sigma"=0.0, "pixel_size"=0.0} ("params"), "Icutoff"=w320, "Isat"=w319, "sigma"=w318, "pixel_size"=w301) -> (w312:T19)
              n161 = Select(t=w308, s=w309, f=w307) -> (s? t:f=w306:u16[][])
              n162 = call <userlib>:"Compute_OD.vi"("dark"=w306, "flat"=w305, "atoms"=w304, "ctx in"=w303, "params"=w312, "identity"=w297, "timeout"="calc timeout") -> ("error out"=w317:errorcluster, "alpha"=w323:dbl, "N"=w321:dbl, "OD"=w322:sgl[][])
              n163 = call <userlib>:"BasicErrorLogger.vi"("error in"=w317) -> ("error out"=w329:errorcluster)  [unwired: 1 in, 1 out]
              n164 = call <vilib>:"Clear Errors.vi"("error in (no error)"=w329) -> ()  [unwired: 6 in, 1 out]
              n165 = local write "alpha"(w323) -> ()
              n166 = call <userlib>:"Set Data Name__ogtk.vi"("Data Name"="atom_number", "Data"=w321) -> ("Renamed Data"=w325:variant)  [unwired: 8 in, 1 out]
              n167 = property class="Clust (strict)"() -> ("Value"=w328:T24)  [unwired: 2 in, 2 out]
              n168 = Build Array(w325) -> (w326:variant[])
              n169 = Bundle(cluster=w328, "sequence"=w331, "name"="OD", "data"=w322, "params"=w326) -> (w300:T24)
              n170 = Build Array (concatenate)(w298, w300) -> (w299:T14)
            }
          }
        }
        "comp_data" <- w243
        n171 = case shown="Default" w252 {
          tunnel: w250 -> [_ w257]
          frame Default {
            n172 = local read "frame"() -> (w256:i32)
            n173 = property on="frame" class="DigNum (strict)"("Val(Sgnl)"=w256) -> ()  [unwired: 2 in, 2 out]
          }
          frame 1.. {
            n174 = property on="comp_list" class="MCListbox (strict)"(error in=w257, "Val(Sgnl)"=0 ("Value (Signaling)")) -> ()  [unwired: 1 in, 2 out]
          }
        }
        n175 = Greater Than 0?(x=w249) -> (x > 0?=w247:bool)
        n176 = for {
          tunnel: w243 -> [w276] mode=indexing
          tunnel: [w275] -> w255 mode=indexing
          n177 = Unbundle(w276) -> ("sequence"=w274:string, "name"=w273:string)  [unwired: 2 out]
          n178 = Build Array(w274, w273) -> (w275:string[])
        }
        n179 = call <userlib>:"GrayOut.vi"("enabled?"=w247) -> ("state"=w248:T21)
        n180 = case shown="True" "histograms" {
          frame False {
          }
          frame True {
            # "Raw image histograms (very slow)"
            n181 = property on="image_data" class="Arr (strict)"() -> ("Value"=w259:u16[][][])  [unwired: 2 in, 2 out]
            n182 = for {
              tunnel: w259 -> [w267] mode=indexing
              tunnel: [w263] -> w260 mode=indexing
              n183 = Array Size(array=w267) -> (size(s)=w269:i32[])
              n184 = Multiply Array Elements(1:w269) -> (0:w268:i32)
              n185 = Reshape Array(w267, w268) -> (w266:u16[])
              n186 = call <vilib>:"General Histogram.vi"("X"=w266, "max"=16384.0, "min"=0.0, "# bins"=400 ("intervals")) -> ("Histogram Graph"=w264:T25)  [unwired: 7 in, 4 out]
              n187 = Bundle("Histogram Graph"=w264) -> (w263:T26)  [unwired: 1 in]
            }
            "raw histograms" <- w260
          }
        }
        n188 = property on="n_atoms" class="DigNum (strict)"("Value"=w249, "DisabledEnum"=w248) -> ()  [unwired: 2 in, 2 out]
        n189 = case shown="True" "auto fit" {
          tunnel: w251 -> [_ w272]
          tunnel: w250 -> [_ w270]
          frame False {
          }
          frame True {
            n190 = Enqueue Element At Opposite End(queue=w272, element=Imaging_State."Fit", error in (no error)=w270) -> ()  [unwired: 1 in, 3 out]
          }
        }
        n191 = property on="comp_list" class="MCListbox (strict)"("ItemNames"=w255) -> ()  [unwired: 2 in, 2 out]
      }
      frame "Fit" {
        n192 = local read "fit_roi"() -> (w369:T10)
        n193 = property on="comp_data" class="Arr (strict)"() -> ("Value"=w348:T14)  [unwired: 2 in, 2 out]
        n194 = local read "frame"() -> (w358:i32)
        n195 = local read "binning"() -> (w335:cluster{"x":u8, "y":u8})
        n196 = property on="image_data" class="Arr (strict)"() -> ("Value"=w349:u16[][][])  [unwired: 2 in, 2 out]
        n197 = local read "roi_capture"() -> (w365:T6)
        n198 = Unbundle By Name(w369) -> ("rect"=w351:T6)
        n199 = Max & Min(x=w358, y=0) -> (max(x,y)=w356:i32)  [unwired: 1 out]
        n200 = Unbundle(w335) -> ("x"=w338:u8, "y"=w339:u8)
        n201 = call <userlib>:"Validate_Rect_Default.vi"("rect"=w351, "default"=w365) -> ("out"=w350:T6)
        n202 = Negate(x=w365) -> (-x=w364:T6)
        n203 = Empty Array?(array=w348) -> (empty?=w362:bool)
        n204 = Bundle("x"=w338, "y"=w339, "x"=w338, "y"=w339) -> (w337:cluster{"x":u8, "y":u8, "x":u8, "y":u8})  [unwired: 1 in]
        n205 = Index Array(array=w348) -> (element=w367:T24)  [unwired: 1 in]
        n206 = Index Array(array=w349, index (dim 0)=w356) -> (element=w359:u16[][])  [unwired: 2 in]
        n207 = Unbundle By Name(w367) -> ("data"=w361:sgl[][])
        n208 = call <userlib>:"Apply_Rect_Offset.vi"("offset rect"=w364, "input"=w350) -> ("output"=w342:T6)  [unwired: 3 in]
        n209 = Quotient & Remainder(x=w342, y=w337) -> (floor(x/y)=w341:T6)  [unwired: 1 out]
        n210 = Select(t=w359, s=w362, f=w361) -> (s? t:f=w360:sgl[][])
        n211 = Unbundle(w341) -> ("left"=w353:i32, "top"=w352:i32, "right"=w375:i32, "bottom"=w374:i32)
        n212 = Multiply(x=w341, y=w337) -> (x*y=w340:T6)
        n213 = Subtract(x=w374, y=w352) -> (x-y=w373:i32)
        n214 = Subtract(x=w375, y=w353) -> (x-y=w372:i32)
        n215 = Array Subset(array=w360, index (row)=w352, length (row)=w373, index (col)=w353, length (col)=w372) -> (w371:sgl[][])
        n216 = local read "fit_function"() -> (w344:enum16{"Gaussian", "ThomasFermi"})
        n217 = Array Size(array=w371) -> (size(s)=w370:i32[])
        n218 = Multiply Array Elements(1:w370) -> (0:w345:i32)
        n219 = Format Into String(w344) -> (resulting string=w343:string)  [unwired: 3 in, 1 out]
        n220 = call <vilib>:"Set Busy.vi"("disable click? (T)"=FALSE) -> ("error out"=w363:errorcluster)  [unwired: 9 in, 1 out]
        n221 = Greater Than 0?(x=w345) -> (x > 0?=w368:bool)
        n222 = case shown="True" w368 {
          tunnel: w371 -> [_ w378]
          tunnel: w340 -> [_ w413]
          tunnel: w363 -> [_ _]
          tunnel: [_ TRUE] -> w355
          tunnel: [errorcluster {"status"=FALSE, "code"=0, "source"=""} ("error in (no error)") _] -> w347
          tunnel: w346 -> [_ w406]
          tunnel: w345 -> [_ w404]
          tunnel: w343 -> [_ w398]
          tunnel: [_ w386] -> w336
          tunnel: [_ w384] -> _
          tunnel: w335 -> [_ w379]
          frame False {
          }
          frame True {
            n223 = Square Root(x=w404) -> (sqrt(x)=w403:dbl)
            n224 = Divide(x=w403, y=200 ("fit_rebin")) -> (x/y=w401:dbl)
            n225 = Round To Nearest(number=w401) -> (nearest integer value=w396:dbl)
            n226 = Max & Min(x=w396, y=1.0) -> (max(x,y)=w394:dbl)  [unwired: 1 out]
            n227 = local read "camera name"() -> (w377:string)
            n228 = local read "calc timeout"() -> (w380:u32)
            n229 = local read "fit clip"() -> (w400:dbl)
            n230 = local write "bin_size"(w394) -> ()
            n231 = call <userlib>:"Compute_Fit.vi"("ctx in"=w406, "rebin_factor"=w394, "timeout"=w380, "data"=w378, "fit_function"=w398, "clip"=w400, "identity"=w377, "binning"=w379) -> ("fit"=w410:variant, "X_section"=→"X-lineout":dbl[][], "Y_section"=→"Y-lineout":dbl[][], "error out"=w420:errorcluster)  [unwired: 4 in]
            n232 = Get Variant Attribute(Variant=w410) -> (duplicate Variant=w409:variant, names=w419:string[])  [unwired: 3 in, 2 out]
            n233 = call <userlib>:"BasicErrorLogger.vi"("error in"=w420) -> ("error out"=w425:errorcluster)  [unwired: 1 in, 1 out]
            n234 = Unbundle By Name(w413) -> ("left"=w414:i32, "top"=w411:i32)
            n235 = for {
              tunnel: [w432] -> w417 mode=indexing
              tunnel: w419 -> [w426] mode=indexing
              tunnel: w409 -> [w431]
              tunnel: dbl[] [] -> [w430]
              n236 = Get Variant Attribute(Variant=w431, name=w426, default value (empty Variant)=w430) -> (value=w429:dbl[])  [unwired: 1 in, 3 out]
              n237 = Index Array(array=w429) -> (element #1=w428:dbl, element #2=w427:dbl)  [unwired: 2 in]
              n238 = Bundle(w426, w428, w427) -> (w432:cluster{string, dbl, dbl})  [unwired: 1 in]
            }
            "fit_params" <- w417
            n239 = call <vilib>:"Clear Errors.vi"("error in (no error)"=w425) -> ()  [unwired: 6 in, 1 out]
            n240 = call <userlib>:"Set Data Name__ogtk.vi"("Data Name"="fit_offset_X", "Data"=w414) -> ("Renamed Data"=w383:variant)  [unwired: 8 in, 1 out]
            n241 = call <userlib>:"Set Data Name__ogtk.vi"("Data Name"="fit_offset_Y", "Data"=w411) -> ("Renamed Data"=w382:variant)  [unwired: 8 in, 1 out]
            n242 = Build Array(w383, w382) -> (w381:variant[])
            n243 = Concatenate Strings(w398, "_Nint" ("Data Name")) -> (w397:string)
            n244 = local read "effective_pixel"() -> (w424:dbl)
            n245 = local read "xsection"() -> (w421:dbl)
            n246 = local read "binning"() -> (w390:cluster{"x":u8, "y":u8})
            n247 = Unbundle(w390) -> ("x"=w389:u8, "y"=w388:u8)
            n248 = Get Variant Attribute(Variant=w409, name=w397, default value (empty Variant)=dbl[] []) -> (value=w408:dbl[], error out=w385:errorcluster)  [unwired: 1 in, 2 out]
            n249 = Square(x=w424) -> (x^2=w423:dbl)
            n250 = Index Array(array=w408) -> (element=w405:dbl)  [unwired: 1 in]
            n251 = Compound Arithmetic op=MULTIPLY(w405, w423, invert w421, w389, w388) -> (w392:dbl)
            "fit_number" <- w392
            n252 = call <userlib>:"Set Data Name__ogtk.vi"("error in (no error)"=w385, "Data Name"="fit_number", "Data"=w392) -> ("error out"=w384:errorcluster, "Renamed Data"=w387:variant)  [unwired: 7 in]
            n253 = Build Array (concatenate)(w387, w381) -> (w386:variant[])
          }
        }
        "fit_current" <- w355
        "fit attribs" <- w336
        n254 = call <vilib>:"Unset Busy.vi"("error in (no error)"=w347) -> ()  [unwired: 10 in, 1 out]
        n255 = property on="fit_buttons" class="Clust (strict)"("Value"=cluster{"selection":bool, "stored":bool} {"selection"=FALSE, "stored"=FALSE} ("fit_buttons")) -> ()  [unwired: 2 in, 2 out]
      }
      frame "Read File" {
        n256 = local write "recent_error"(FALSE ("recent_error")) -> ()
        n257 = local read "working dir"() -> (w438:path)
        n258 = local read "current file"() -> (w437:string)
        n259 = property on="continuous" class="Bool (strict)"("Value"=FALSE ("continuous")) -> ()  [unwired: 2 in, 2 out]
        n260 = case shown="Default" w437 {
          selector: w437 -> [w471 _]
          tunnel: w439 -> [w442 _]
          tunnel: w438 -> [w472 _]
          tunnel: w434 -> [w457 _]
          tunnel: w433 -> [w440 _]
          frame Default {
            n261 = local read "camera name"() -> (w474:string)
            n262 = Build Path(base path=w472, name or relative path=w471) -> (appended path=w452:path)
            n263 = Path To String(path=w452) -> (string=w458:string)
            n264 = call-dynamic "ZLockAcquire.vi"("key"=w458, "ZLock in"=w457) -> ("error out"=w451:errorcluster, "key out"=w455:string, "ZLock out"=w456:refnum<class "ZLock.lvclass">)  [unwired: 7 in]
            n265 = Concatenate Strings("Read file  " ("text"), w471) -> (w476:string)
            n266 = call <vilib>:"H5Fopen.vi"("error in (no error)"=w451, "mode (read-only)"=H5Fmode."read-only", "path"=w452) -> ("error out"=w447:errorcluster, "ref out"=w450:T27)  [unwired: 7 in]
            n267 = Concatenate Strings("/devices/" ("Name"), w474) -> (w446:string)
            n268 = call <userlib>:"BasicLogger.vi"("text"=w476) -> ()  [unwired: 6 in, 2 out]
            n269 = call <vilib>:"H5Gopen.vi"("error in (no error)"=w447, "name"=w446, "ref in"=w450) -> ("error out"=w448:errorcluster, "group out"=w449:T27)  [unwired: 7 in]
            n270 = case shown="No Error" w448 {
              selector: w448 -> [_ w659]
              tunnel: [w541 w658] -> w445
              tunnel: w449 -> [w531 _]
              tunnel: [w515 w661] -> w444
              tunnel: [w540 w656] -> w464
              tunnel: [w534 w657] -> w467
              tunnel: [w537 w662] -> w466
              tunnel: w450 -> [w514 w661]
              frame No Error {
                w503 = string[] []
                w500 = "EXPOSURES" ("name")
                # "When is the experiment scheduled to finish?"
                n271 = xnode "H5Aread.xnode"("default"=0.0, "attrib name"="exposure_time" ("attribute"), "ref in"=w531) -> ("error out"=w525:errorcluster, "data"=w528:dbl, "ref out"=w527:T27)  [unwired: 3 in, 1 out]
                n272 = Multiply(x=w528, y=1000.0) -> (x*y=w542:dbl)
                n273 = local write "exposure"(w542) -> ()
                n274 = xnode "H5Aread.xnode"("error in (no error)"=w525, "default"="", "attrib name"="orientation" ("attribute"), "ref in"=w527) -> ("error out"=w509:errorcluster, "data"=w523:string, "ref out"=w508:T27)  [unwired: 2 in, 1 out]
                "location" <- w523
                n275 = Concatenate Strings("/images/" ("Name"), w523) -> (w521:string)
                n276 = xnode "H5Aread.xnode"("object name"="/devices/pulseblaster_0" ("Name"), "default"=0.0, "attrib name"="stop_time" ("attribute"), "ref in"=w514) -> ("error out"=w516:errorcluster, "data"=w510:dbl, "ref out"=w515:T27)  [unwired: 2 in, 1 out]
                n277 = xnode "H5Dread.xnode"("type name (default)"="frametype", "dataset name (this)"=w500, "error in (no error)"=w509, "default"=w503, "ref in"=w508) -> ("error out"=w502:errorcluster, "data"=w507:string[], "ref out"=w506:T27)  [unwired: 1 in, 1 out]
                n278 = case shown="No Error" w516 {
                  tunnel: w510 -> [w655 _]
                  frame No Error {
                    "stop_time" <- w655
                  }
                  frame Error {
                  }
                }
                n279 = xnode "H5Dread.xnode"("type name (default)"="name", "dataset name (this)"=w500, "error in (no error)"=w502, "default"=w503, "ref in"=w506) -> ("error out"=w501:errorcluster, "data"=w504:string[], "ref out"=w505:T27)  [unwired: 1 in, 1 out]
                n280 = call <vilib>:"H5Gclose.vi"("error in (no error)"=w501, "group in"=w505) -> ("error out"=w522:errorcluster)  [unwired: 9 in]
                n281 = property on="image_data" class="Arr (strict)"() -> ("Value"=w533:u16[][][])  [unwired: 2 in, 2 out]
                n282 = call <vilib>:"H5Lexists.vi"("error in (no error)"=w522, "path"=w521, "ref in"=w514) -> ("error out"=w520:errorcluster, "exists?"=w518:bool, "path out"=w519:string, "ref out"=w517:T27)  [unwired: 5 in]
                n283 = property on="raw_list" class="MCListbox (strict)"() -> ("ItemNames"=w539:string[][])  [unwired: 2 in, 2 out]
                n284 = call <userlib>:"Fix Sequence.vi"("sequences"=w504, "shots"=w507, "old sequence list"=w539, "image_data"=w533, "keep?"="hold_frames") -> ("sequencer"=w537:T28, "held data"=w536:u16[][][])
                n285 = case shown="True" w518 {
                  tunnel: [w619 w627] -> w541
                  tunnel: w519 -> [_ w631]
                  tunnel: [_ w639] -> w540
                  tunnel: [_ w638] -> w535
                  tunnel: w517 -> [_ w632]
                  tunnel: w520 -> [w619 w630]
                  tunnel: w537 -> [_ w634]
                  frame False {
                    # "Group doesn't exist yet, this is a new shot"
                  }
                  frame True {
                    n286 = call <vilib>:"H5Gopen.vi"("error in (no error)"=w630, "name"=w631, "ref in"=w632) -> ("error out"=w625:errorcluster, "group out"=w626:T27)  [unwired: 7 in]
                    n287 = xnode "H5Aread.xnode"("error in (no error)"=w625, "default"=u8[] [1, 1], "attrib name"="binning" ("attrib_name"), "ref in"=w626) -> ("error out"=w624:errorcluster, "data"=w622:u8[], "ref out"=w623:T27)  [unwired: 2 in, 1 out]
                    n288 = Array To Cluster(array=w622) -> (cluster=w633:cluster{"data[0]":u8, "data[1]":u8})
                    n289 = call <userlib>:"Read_Exposures.vi"("ref in"=w623, "sequencer"=w634, "error in"=w624) -> ("ref out"=w629:i32, "ROI"=w637:T6, "loaded images"=w638:u16[][][], "computations"=w639:T29, "error out"=w628:errorcluster)  [unwired: 1 in]
                    n290 = local read "roi_capture"() -> (w636:T6)
                    n291 = local write "binning"(w633) -> ()
                    n292 = call <userlib>:"Validate_Rect_Default.vi"("rect"=w637, "default"=w636) -> ("out"=w635:T6)
                    n293 = local write "roi_capture"(w635) -> ()
                    n294 = call <vilib>:"H5Gclose.vi"("error in (no error)"=w628, "group in"=w629) -> ("error out"=w627:errorcluster)  [unwired: 9 in]
                  }
                }
                n295 = Build Array (concatenate)(w536, w535) -> (w534:u16[][][])
              }
              frame Error {
                n296 = Greater Than 0?(x=w661) -> (x > 0?=w660:bool)
                n297 = case shown="True" w660 {
                  tunnel: w659 -> [w664 _]
                  tunnel: [w664 w667] -> w658
                  frame False {
                  }
                  frame True {
                    n298 = local read "camera name"() -> (w665:string)
                    n299 = Concatenate Strings("Specified HDF has no instructions for camera " ("error message (\"\")"), w665) -> (w666:string)
                    n300 = call <vilib>:"Error Cluster From Error Code.vi"("error message (\"\")"=w666, "error code (0)"=6013) -> ("error out"=w667:errorcluster)  [unwired: 7 in]
                  }
                }
                n301 = local write "current file"("") -> ()
                n302 = property on="comp_data" class="Arr (strict)"() -> ("Value"=w656:T14)  [unwired: 2 in, 2 out]
                n303 = local read "sequencer"() -> (w662:T13)
                n304 = property on="image_data" class="Arr (strict)"() -> ("Value"=w657:u16[][][])  [unwired: 2 in, 2 out]
              }
            }
            "sequencer" <- w466
            n305 = call <vilib>:"H5Fclose.vi"("error in (no error)"=w445, "ref"=w444) -> ("error out"=w441:errorcluster)  [unwired: 9 in]
            n306 = local write "image_data"(w467) -> ()
            n307 = local write "comp_data"(w464) -> ()
            n308 = for {
              tunnel: [w479] -> w465 mode=indexing
              tunnel: w464 -> [w477] mode=indexing
              n309 = Unbundle(w477) -> ("sequence"=w480:string, "name"=w478:string)  [unwired: 2 out]
              n310 = Build Array(w480, w478) -> (w479:string[])
            }
            n311 = Lossy Enqueue Element(queue=w440, element=w441) -> ()  [unwired: 1 in, 4 out]
            n312 = case shown="Error" w441 {
              tunnel: [w494 w497] -> _
              tunnel: w442 -> [w494 w496]
              frame No Error {
              }
              frame Error {
                n313 = local write "current file"("") -> ()
                n314 = Flush Queue(queue=w496) -> (queue out=w497:refnum<queue>)  [unwired: 1 in, 2 out]
              }
            }
            n315 = for {
              tunnel: w466 -> [w490] mode=indexing
              tunnel: [w487] -> w463 mode=indexing
              shift-right: [w484] -> w462
              shift-left: string[][] [] -> [w483]
              n316 = Unbundle(w490) -> ("name"=w485:string, "shots"=w486:string[])  [unwired: 1 out]
              n317 = Equal?(x=w485, y="(held)") -> (x = y?=w488:bool)
              n318 = for {
                tunnel: w486 -> [w493] mode=indexing
                tunnel: w485 -> [w492]
                tunnel: [w491] -> w482 mode=indexing
                n319 = Build Array(w492, w493) -> (w491:string[])
              }
              n320 = Boolean To (0,1)(Boolean=w488) -> (0, 1=w487:i16)
              n321 = Build Array (concatenate)(w482, w483) -> (w484:string[][])
            }
            n322 = call <vilib>:"Clear Errors.vi"("error in (no error)"=w441) -> ("error out"=w454:errorcluster)  [unwired: 6 in]
            n323 = Merge Errors(w451, w454) -> (w453:errorcluster)
            n324 = call-dynamic "ZLockRelease.vi"("error in (no error)"=w453, "key"=w455, "ZLock in"=w456) -> ()  [unwired: 6 in, 3 out]
            n325 = local write "fit_current"(FALSE ("fit_current")) -> ()
            n326 = Array Size(array=w464) -> (size(s)=w469:i32)
            n327 = property on="comp_list" class="MCListbox (strict)"("ItemNames"=w465) -> ()  [unwired: 2 in, 2 out]
            n328 = Greater Than 0?(x=w469) -> (x > 0?=w468:bool)
            n329 = case shown="True" w468 {
              frame False {
              }
              frame True {
                n330 = property on="comp_list" class="MCListbox (strict)"("Val(Sgnl)"=0 ("display_frame")) -> ()  [unwired: 2 in, 2 out]
              }
            }
            n331 = property on="n_atoms" class="DigNum (strict)"("DisabledEnum"=T21."Enabled" ("Disabled")) -> ()  [unwired: 2 in, 2 out]
            n332 = Add Array Elements(numeric array=w463) -> (sum=→"keep":i16)
            n333 = property on="raw_list" class="MCListbox (strict)"("ItemNames"=w462) -> ()  [unwired: 2 in, 2 out]
          }
          frame "" {
            n334 = call <userlib>:"BasicLogger.vi"("text"="Empty \"read file\" command") -> ()  [unwired: 6 in, 2 out]
          }
        }
      }
      frame "Save File" {
        n335 = local read "working dir"() -> (w676:path)
        n336 = local read "current file"() -> (w675:string)
        n337 = Get Queue Status(queue=w673) -> ()  [unwired: 2 in, 8 out]
        n338 = case shown="Default" w675 {
          selector: w675 -> [w695 _]
          tunnel: w676 -> [w696 _]
          tunnel: [w684 w791] -> w671
          tunnel: w674 -> [w691 _]
          tunnel: [w689 _] -> _
          frame Default {
            n339 = Build Path(base path=w696, name or relative path=w695) -> (appended path=w687:path)
            n340 = Path To String(path=w687) -> (string=w694:string)
            n341 = local read "location"() -> (w698:string)
            n342 = call-dynamic "ZLockAcquire.vi"("key"=w694, "ZLock in"=w691) -> ("error out"=w686:errorcluster, "key out"=w692:string, "ZLock out"=w690:refnum<class "ZLock.lvclass">)  [unwired: 7 in]
            n343 = Concatenate Strings("Save file  " ("text"), w695) -> (w699:string)
            n344 = call <vilib>:"H5Fopen.vi"("error in (no error)"=w686, "mode (read-only)"=H5Fmode."read-write", "path"=w687) -> ("error out"=w678:errorcluster, "ref out"=w683:T27)  [unwired: 7 in]
            n345 = Concatenate Strings("images/" ("attribute"), w698) -> (w682:string)
            n346 = call <userlib>:"BasicLogger.vi"("text"=w699) -> ()  [unwired: 6 in, 2 out]
            n347 = call <vilib>:"H5Gopen.vi"("create? (F)"=TRUE, "error in (no error)"=w678, "name"=w682, "ref in"=w683) -> ("error out"=w681:errorcluster, "group out"=w680:T27)  [unwired: 6 in]
            n348 = case shown="No Error" w681 {
              selector: w681 -> [_ w788]
              tunnel: [w713 w788] -> w685
              tunnel: w680 -> [w711 _]
              frame No Error {
                n349 = property on="rois" class="Arr (strict)"() -> ("Value"=w710:T7)  [unwired: 2 in, 2 out]
                n350 = local read "effective_pixel"() -> (w720:dbl)
                n351 = local read "camera name"() -> (w724:string)
                n352 = for {
                  tunnel: w711 -> [w760]
                  tunnel: w710 -> [w752] mode=indexing
                  tunnel: [w758] -> w701
                  shift-right: [w757] -> w709
                  shift-left: _ -> [w756]
                  i -> [w755]
                  n353 = Unbundle(w752) -> ("rect"=w751:T6)  [unwired: 3 out]
                  n354 = Format Into String(format string="roi%d", w755) -> (resulting string=w753:string)  [unwired: 2 in, 1 out]
                  n355 = call <userlib>:"Validate_Rect.vi"("rect"=w751) -> ("valid"=w750:bool)
                  n356 = case shown="True" w750 {
                    tunnel: w760 -> [w762 w769]
                    tunnel: TRUE ("overwrite? (F)") -> [_ w765]
                    tunnel: [w762 w763] -> w758
                    tunnel: [w761 w764] -> w757
                    tunnel: w756 -> [w761 w768]
                    tunnel: w753 -> [_ w766]
                    tunnel: w751 -> [_ w767]
                    frame False {
                    }
                    frame True {
                      n357 = xnode "H5Awrite.xnode"("replace? (T)"=w765, "error in (no error)"=w768, "data"=w767, "attrib name"=w766, "ref in"=w769) -> ("error out"=w764:errorcluster, "ref out"=w763:T27)  [unwired: 2 in, 1 out]
                    }
                  }
                }
                n358 = local read "attribs"() -> (w722:variant[])
                n359 = call <userlib>:"Set Data Name__ogtk.vi"("Data Name"="effective_pixel_size", "Data"=w720) -> ("Renamed Data"=w718:variant)  [unwired: 8 in, 1 out]
                n360 = call <userlib>:"Set Data Name__ogtk.vi"("Data Name"="camera", "Data"=w724) -> ("Renamed Data"=w721:variant)  [unwired: 8 in, 1 out]
                n361 = Build Array (concatenate)(w718, w722, w721) -> (w703:variant[])
                n362 = for {
                  tunnel: w703 -> [w729] mode=indexing
                  tunnel: [w730] -> w704
                  shift-right: [w731] -> w702
                  shift-left: w701 -> [w725]
                  n363 = call <userlib>:"Get Data Name__ogtk.vi"("Data"=w729) -> ("Data Name"=w727:string, "Data dup"=w728:variant)  [unwired: 8 in, 1 out]
                  n364 = call <vilib>:"H5Awrite_var.vi"("replace? (T)"=FALSE ("overwrite?"), "data"=w728, "attrib name"=w727, "ref in"=w725) -> ("error out"=w730:errorcluster, "ref out"=w731:T27)  [unwired: 5 in, 1 out]
                }
                n365 = property on="sequencer" class="Arr (strict)"() -> ("Value"=w707:T13)  [unwired: 2 in, 2 out]
                n366 = property on="image_data" class="Arr (strict)"() -> ("Value"=w708:u16[][][])  [unwired: 2 in, 2 out]
                n367 = call <vilib>:"Clear Errors.vi"("error in (no error)"=w704) -> ()  [unwired: 6 in, 1 out]
                n368 = local read "fit_current"() -> (w712:bool)
                n369 = property on="comp_data" class="Arr (strict)"() -> ("Value"=w706:T14)  [unwired: 2 in, 2 out]
                n370 = call <userlib>:"Write_raw_data.vi"("image_data"=w708, "sequencer"=w707, "ref in"=w702) -> ("error out"=w714:errorcluster, "ref out"=w717:i32)  [unwired: 3 in]
                n371 = case shown="True" "Save OD" {
                  tunnel: w717 -> [_ w736]
                  tunnel: [_ w735] -> w716
                  tunnel: [_ w734] -> w715
                  tunnel: w712 -> [_ w733]
                  tunnel: w706 -> [_ w732]
                  frame False {
                  }
                  frame True {
                    n372 = call <userlib>:"Write_comp_data.vi"("comp_data"=w732, "ref in"=w736) -> ("error out"=w734:errorcluster, "ref out"=w737:i32)  [unwired: 2 in]
                    n373 = case shown="True" w733 {
                      tunnel: w732 -> [_ w740]
                      tunnel: w737 -> [_ w739]
                      tunnel: [_ w738] -> w735
                      frame False {
                      }
                      frame True {
                        n374 = for {
                          tunnel: w740 -> [w749] mode=indexing
                          tunnel: w739 -> [w744]
                          tunnel: [w742] -> w738 mode=indexing
                          n375 = Unbundle By Name(w749) -> ("sequence"=w748:string, "name"=w747:string)
                          n376 = local read "fit_params"() -> (w741:T9)
                          n377 = local read "fit attribs"() -> (w745:variant[])
                          n378 = Concatenate Strings(w748, "/" ("string"), w747) -> (w743:string)
                          n379 = call <userlib>:"Write_fit_data.vi"("dset name"=w743, "fit attribs"=w745, "fit_params"=w741, "ref in"=w744) -> ("error out"=w742:errorcluster)  [unwired: 3 in, 1 out]
                        }
                      }
                    }
                  }
                }
                n380 = Merge Errors(w716, w715, w714, w709) -> (w713:errorcluster)
              }
              frame Error {
              }
            }
            n381 = call <vilib>:"H5Fclose.vi"("error in (no error)"=w685, "ref"=w683) -> ("error out"=w684:errorcluster)  [unwired: 9 in]
            n382 = call <vilib>:"Clear Errors.vi"("error in (no error)"=w684) -> ("error out"=w693:errorcluster)  [unwired: 6 in]
            n383 = Merge Errors(w686, w693) -> (w688:errorcluster)
            n384 = call-dynamic "ZLockRelease.vi"("error in (no error)"=w688, "key"=w692, "ZLock in"=w690) -> ("error out"=w689:errorcluster)  [unwired: 6 in, 2 out]
          }
          frame "" {
            n385 = call <vilib>:"Error Cluster From Error Code.vi"("error message (\"\")"="Cannot save file - no filename specified" ("error message (\"\")"), "error code (0)"=6015) -> ("error out"=w791:errorcluster)  [unwired: 7 in]
          }
        }
        n386 = Lossy Enqueue Element(queue=w672, element=w671) -> ()  [unwired: 1 in, 4 out]
      }
    }
  }
  n387 = while {
    tunnel: w24 -> [w793]
    tunnel: w36 -> [w794]
    stop <- FALSE stop-if-true
    n388 = event shown="[4] \"files\": Value Change" {
      selector: _ -> [_ _ _ _ _ _ _ _ _ _ _ _ _ _ _ _ _]
      dyn-events: _ -> [_ _ _ _ _ _ _ _ _ _ _ _ _ _ _ _ _]
      timeout: 200 -> [_ _ _ _ _ _ _ _ _ _ _ _ _ _ _ _ _]
      tunnel: w794 -> [_ _ _ w829 w832 w875 _ _ w945 w965 _ _ _ _ _ _ _]
      tunnel: w793 -> [w796 _ _ _ _ w874 _ _ w944 _ _ _ _ _ _ _ _]
      event Timeout {
        w798 = 4 items=["None", "Selection Tool", "Point Tool", "Line Tool", "Rectangle Tool", "Oval Tool", "Polygon Tool", "ClosedFreehandTool", "Annulus Tool", "Rotated Rectangle Tool", "Zoom Tool", "Pan Tool", "Polyline Tool", "Freehand Tool"] ("Tool")
        n389 = event-data() -> ()  [unwired: 1 in, 2 out]
        n390 = invoke on="img_OD" class="ImageControl" method="Get Last Event"("Which Events"=i32[] [2, 1]) -> ("Tool"=w799:i32)  [unwired: 7 in, 7 out]
        n391 = Equal?(x=w799, y=w798) -> (x = y?=w797:bool)
        n392 = case shown="True" w797 {
          tunnel: w796 -> [_ _]
          frame False {
          }
          frame True {
            n393 = local read "binning"() -> (w801:cluster{"x":u8, "y":u8})
            n394 = property on="img_OD" class="ImageControl"() -> ("ROI"=w807:T32)  [unwired: 2 in, 2 out]
            n395 = call <userlib>:"ROI_to_rects.vi"("binning"=w801, "ROI"=w807) -> ("rect"=w806:T6)  [unwired: 3 out]
            n396 = local read "roi_capture"() -> (w805:T6)
            n397 = local read "roi_capture"() -> (w803:T6)
            n398 = call <userlib>:"Apply_Rect_Offset.vi"("offset rect"=w805, "input"=w806) -> ("output"=w804:T6)  [unwired: 3 in]
            n399 = call <userlib>:"Clip_Rect.vi"("bounds"=w803, "rect"=w804) -> ("result"=w802:T6)  [unwired: 1 in]
            n400 = property on="roi_current" class="Clust (strict)"("Val(Sgnl)"=w802) -> ()  [unwired: 2 in, 2 out]
          }
        }
      }
      event "newinst": Value Change {
        # "Doesn't appear to actually \"run\" the clone"
        n401 = event-data() -> ("NewVal"=w808:bool)  [unwired: 1 in, 4 out]
        n402 = case shown="True" w808 {
          tunnel: [_ w812] -> _
          frame False {
          }
          frame True {
            n403 = property class="VI"() -> ("Path"=w820:path)  [unwired: 2 in, 2 out]
            n404 = Open VI Reference(vi path=w820, options=8) -> (vi reference=w816:refnum<vi>)  [unwired: 4 in, 1 out]
            n405 = invoke class="VI" method="FP.Open"(reference=w816, "Activate"=TRUE ("Activate?"), "State"=T30."Maximized") -> (reference out=w818:refnum<vi>, error out=w817:errorcluster)  [unwired: 2 in, 3 out]
            n406 = invoke class="VI" method="Run VI"(reference=w818, error in=w817, "Wait until done"=FALSE ("Wait Until Done")) -> (reference out=w814:refnum<vi>, error out=w815:errorcluster)  [unwired: 2 in, 3 out]
            n407 = local write "newinst"(FALSE ("newinst")) -> ()
            n408 = Close Reference(reference=w814, error in (no error)=w815) -> (error out=w812:errorcluster)
          }
        }
      }
      event Value Change {
        # "Something with interrupts to improve flicker"
        n409 = event-data() -> ()  [unwired: 1 in, 5 out]
        n410 = local read "roi_capture"() -> (w826:T6)
        n411 = local read "roi_current"() -> (w822:T6)
        n412 = Negate(x=w826) -> (-x=w825:T6)
        n413 = local read "binning"() -> (w821:cluster{"x":u8, "y":u8})
        n414 = call <userlib>:"Apply_Rect_Offset.vi"("offset rect"=w825, "input"=w822) -> ("output"=w824:T6)  [unwired: 3 in]
        n415 = call <userlib>:"Rect_to_ROI.vi"("rect"=w824, "binning"=w821) -> ("ROI"=w823:T33)
        n416 = property on="img_OD" class="ImageControl"("ROI"=w823) -> ()  [unwired: 2 in, 2 out]
      }
      event "stop": Value Change {
        n417 = event-data() -> ()  [unwired: 1 in, 5 out]
        n418 = Flush Queue(queue=w829) -> (queue out=w827:refnum<queue>)  [unwired: 1 in, 2 out]
        n419 = Enqueue Element(queue=w827, element=Imaging_State."Quit") -> ()  [unwired: 2 in, 3 out]
      }
      event "files": Value Change {
        n420 = event-data() -> ("OldVal"=w834:T1, "NewVal"=w833:T1)  [unwired: 1 in, 3 out]
        n421 = Cluster To Array(cluster=w834) -> (array=w836:bool[])
        n422 = Cluster To Array(cluster=w833) -> (array=w835:bool[])
        n423 = call <userlib>:"Detect_Boolean_Change.vi"("NewVal"=w835, "OldVal"=w836) -> ("ButtonId"=w831:i32)  [unwired: 2 out]
        n424 = Greater Or Equal To 0?(x=w831) -> (x >= 0?=w830:bool)
        n425 = case shown="True" w830 {
          tunnel: w832 -> [_ w837]
          tunnel: w831 -> [_ w838]
          frame False {
          }
          frame True {
            n426 = local read "current file"() -> (w839:string)
            n427 = case shown="0, 1" w838 {
              selector: w838 -> [_ _ _ w848]
              tunnel: w839 -> [_ _ _ w854]
              tunnel: w837 -> [w840 w842 _ w849]
              frame 2 {
                n428 = Enqueue Element(queue=w840, element=Imaging_State."Save File") -> ()  [unwired: 2 in, 3 out]
              }
              frame 3 {
                n429 = Enqueue Element(queue=w842, element=Imaging_State."Compute") -> ()  [unwired: 2 in, 3 out]
              }
              frame Default {
              }
              frame 0, 1 {
                n430 = local read "working dir"() -> (w853:path)
                n431 = call "File Dialog"("start path"=w853, "prompt"="Select H5 File", "default name"=w854, "pattern (all files)"="*.h5", "pattern label"="HDF files") -> ("selected path"=w847:path, "error out"=w845:errorcluster)  [unwired: 7 in, 2 out]
                n432 = call <vilib>:"H5Fis_hdf.vi"("error in (no error)"=w845, "path in"=w847) -> ("error out"=w844:errorcluster, "valid?"=w846:bool)  [unwired: 6 in, 2 out]
                n433 = case shown="False" w846 {
                  tunnel: w847 -> [_ w867]
                  tunnel: w849 -> [_ w866]
                  tunnel: w848 -> [_ w856]
                  tunnel: w844 -> [_ _]
                  frame False {
                    n434 = One Button Dialog(message="Chosen file is not a valid HDF5") -> ()  [unwired: 1 in, 1 out]
                  }
                  frame True {
                    n435 = Flush Queue(queue=w866) -> (queue out=w862:refnum<queue>, remaining elements=w865:T11[])  [unwired: 1 in, 1 out]
                    n436 = Strip Path(path=w867) -> (stripped path=w864:path, name=w863:string)
                    n437 = property on="working dir" class="Path"("Value"=w864) -> (error out=w859:errorcluster)  [unwired: 2 in, 1 out]
                    n438 = Array Size(array=w865) -> (size(s)=w857:i32)
                    n439 = property on="current file" class="Str"(error in=w859, "Value"=w863) -> (error out=w858:errorcluster)  [unwired: 1 in, 1 out]
                    n440 = Enqueue Element(queue=w862, element=Imaging_State."Read File", error in (no error)=w858) -> (queue out=w860:refnum<queue>)  [unwired: 1 in, 2 out]
                    n441 = case shown="Default" w857 {
                      frame 0 {
                      }
                      frame Default {
                        n442 = call <userlib>:"BasicLogger.vi"("text"="File open forced queue clear") -> ()  [unwired: 6 in, 2 out]
                      }
                    }
                    n443 = case shown="Default" w856 {
                      tunnel: w860 -> [w870 w871]
                      frame Default {
                        n444 = Enqueue Element(queue=w870, element=Imaging_State."Redraw") -> ()  [unwired: 2 in, 3 out]
                      }
                      frame 1 {
                        n445 = Enqueue Element(queue=w871, element=Imaging_State."Acquire") -> ()  [unwired: 2 in, 3 out]
                      }
                    }
                  }
                }
              }
            }
          }
        }
      }
      event "capture.abort": Value Change {
        n446 = event-data() -> ("NewVal"=w873:bool)  [unwired: 1 in, 4 out]
        n447 = case shown="True" w873 {
          tunnel: w875 -> [_ w880]
          tunnel: w874 -> [_ w879]
          tunnel: [_ w876] -> _
          frame False {
          }
          frame True {
            n448 = Flush Queue(queue=w880) -> (error out=w877:errorcluster)  [unwired: 1 in, 2 out]
            n449 = call-dynamic "CameraAbort.vi"("error in (no error)"=w877, "CameraBase in"=w879) -> ("error out"=w876:errorcluster)  [unwired: 8 in, 1 out]
            n450 = call <userlib>:"BasicLogger.vi"("text"="Abort signalled") -> ()  [unwired: 6 in, 2 out]
          }
        }
      }
      event "tools_zoom": Value Change {
        n451 = event-data() -> ("OldVal"=w884:T2, "NewVal"=w883:T2)  [unwired: 1 in, 3 out]
        n452 = control-ref of="img_OD"() -> (w881:refnum<vi>)
        n453 = Cluster To Array(cluster=w884) -> (array=w885:bool[])
        n454 = Cluster To Array(cluster=w883) -> (array=w886:bool[])
        n455 = call <userlib>:"Detect_Boolean_Change.vi"("NewVal"=w886, "OldVal"=w885) -> ("ButtonId"=w887:i32)  [unwired: 2 out]
        n456 = Build Array(w881) -> (w882:refnum<vi>[])
        n457 = for {
          tunnel: w887 -> [w889]
          tunnel: [w888] -> _ mode=indexing
          tunnel: w882 -> [w888] mode=indexing
          n458 = case shown="1" w889 {
            tunnel: w888 -> [w890 w908 w920 w928 _]
            frame 0 {
              n459 = property on="Property Node" class="ImageControl" props=["ROI", "Image Area Size", "Image Area Height", "Image Area Width"](reference=w890) -> (reference out=w891:refnum<vi>, "ROI"=w897:T32, "Image Area Height"=w896:u32, "Image Area Width"=w895:u32)  [unwired: 1 in, 2 out]
              n460 = Unbundle(w897) -> ("Global Rectangle"=w894:i32[], "Contours"=w893:T34)
              n461 = Empty Array?(array=w893) -> (empty?=w892:bool)
              n462 = case shown="False" w892 {
                tunnel: w896 -> [w906 _]
                tunnel: w895 -> [w905 _]
                tunnel: w894 -> [w902 _]
                tunnel: w891 -> [w898 _]
                frame False {
                  n463 = formula code="Zx=W/(R[2]-R[0]);\nZy=H/(R[3]-R[1]);\nCx=(R[2]+R[0])/2;\nCy=(R[3]+R[1])/2;"("R"=w902, "H"=w906, "W"=w905) -> ("Zx"=w900:dbl, "Zy"=w901:dbl, "Cx"=w904:dbl, "Cy"=w903:dbl)
                  n464 = Max & Min(x=w900, y=w901) -> (min(x,y)=w899:dbl)  [unwired: 1 out]
                  n465 = property on="Property Node" class="ImageControl"(reference=w898, "X Zoom"=w899, "Y Zoom"=w899, "Image Center X Position"=w904, "Image Center Y Position"=w903) -> ()  [unwired: 1 in, 2 out]
                }
                frame True {
                }
              }
            }
            frame 1 {
              w915 = sgl 1.2 ("x")
              # "Zoom to ROI if possible"
              n466 = property on="Property Node" class="ImageControl"(reference=w908) -> (reference out=w909:refnum<vi>, "X Zoom"=w916:sgl, "Y Zoom"=w917:sgl, "ROI"=w914:T32, "Image Center Position"=w910:cluster{"X":u32, "Y":u32})  [unwired: 1 in, 1 out]
              n467 = local read "binning"() -> (w907:cluster{"x":u8, "y":u8})
              n468 = call <userlib>:"ROI_to_rects.vi"("binning"=w907, "ROI"=w914) -> ("center"=w912:cluster{"x":i16, "y":i16}, "valid"=w913:bool)  [unwired: 2 out]
              n469 = Select(t=w912, s=w913, f=w910) -> (s? t:f=w911:cluster{"X":u32, "Y":u32})
              n470 = Multiply(x=w916, y=w915) -> (x*y=w919:sgl)
              n471 = Multiply(x=w917, y=w915) -> (x*y=w918:sgl)
              n472 = property on="Property Node" class="ImageControl"(reference=w909, "X Zoom"=w919, "Y Zoom"=w918, "Image Center Position"=w911) -> ()  [unwired: 1 in, 2 out]
            }
            frame 2 {
              w922 = sgl 1.2 ("x")
              n473 = property on="Property Node" class="ImageControl"(reference=w920) -> (reference out=w921:refnum<vi>, "X Zoom"=w924:sgl, "Y Zoom"=w925:sgl, "Image Center Position"=w923:cluster{"X":u32, "Y":u32})  [unwired: 1 in, 1 out]
              n474 = Divide(x=w924, y=w922) -> (x/y=w927:sgl)
              n475 = Divide(x=w925, y=w922) -> (x/y=w926:sgl)
              n476 = property on="Property Node" class="ImageControl"(reference=w921, "X Zoom"=w927, "Y Zoom"=w926, "Image Center Position"=w923) -> ()  [unwired: 1 in, 2 out]
            }
            frame 3 {
              n477 = property on="Property Node" class="ImageControl"(reference=w928, "Zoom to Fit Mode"=TRUE) -> ()  [unwired: 1 in, 2 out]
            }
            frame Default {
            }
          }
        }
      }
      event "tools_view": Value Change {
        n478 = event-data() -> ("OldVal"=w932:cluster{"sel":bool, "in":bool, "out":bool}, "NewVal"=w931:cluster{"sel":bool, "in":bool, "out":bool})  [unwired: 1 in, 3 out]
        n479 = Cluster To Array(cluster=w932) -> (array=w939:bool[])
        n480 = Cluster To Array(cluster=w931) -> (array=w938:bool[])
        n481 = call <userlib>:"Detect_Boolean_Change.vi"("NewVal"=w938, "OldVal"=w939) -> ("FinalVal"=w936:bool[], "SingleEvent"=w934:bool, "ButtonId"=w937:i32)
        n482 = Array To Cluster(array=w936) -> (cluster=w933:T35)
        n483 = Select(t=w933, s=w934, f=w932) -> (s? t:f=w930:cluster{"sel":bool, "in":bool, "out":bool})
        n484 = case shown="0" w937 {
          tunnel: [w940 w941 w942 w943] -> w935
          frame Default {
            n485 = property on="img_OD" class="ImageControl"() -> ("Current ROI Tool"=w940:u32)  [unwired: 2 in, 2 out]
          }
          frame 0 {
            w941 = u32 8 items=["No Selection", "Point", "Line", "Rectangle", "Oval", "Polygon", "Freehand Region", "Annulus", "Zoom", "Pan", "Broken Line", "Freehand Line", "Rotated Rectangle"] ("Tool (Point)")
          }
          frame 1 {
            w942 = u32 3 items=["No Selection", "Point", "Line", "Rectangle", "Oval", "Polygon", "Freehand Region", "Annulus", "Zoom", "Pan", "Broken Line", "Freehand Line", "Rotated Rectangle"] ("Tool (Point)")
          }
          frame 2 {
            w943 = u32 9 items=["No Selection", "Point", "Line", "Rectangle", "Oval", "Polygon", "Freehand Region", "Annulus", "Zoom", "Pan", "Broken Line", "Freehand Line", "Rotated Rectangle"] ("Tool (Point)")
          }
        }
        n486 = local write "tools_view"(w930) -> ()
        n487 = property on="img_OD" class="ImageControl"("Current ROI Tool"=w935) -> ()  [unwired: 2 in, 2 out]
      }
      event "capture": Value Change {
        n488 = event-data() -> ("OldVal"=w946:T3, "NewVal"=w947:T3)  [unwired: 1 in, 3 out]
        n489 = Cluster To Array(cluster=w946) -> (array=w950:bool[])
        n490 = Cluster To Array(cluster=w947) -> (array=w949:bool[])
        n491 = call <userlib>:"Detect_Boolean_Change.vi"("NewVal"=w949, "OldVal"=w950) -> ("ButtonId"=w948:i32)  [unwired: 2 out]
        n492 = case shown="0, 1" w948 {
          selector: w948 -> [w959 _]
          tunnel: w945 -> [w955 _]
          tunnel: w944 -> [w953 _]
          frame 0, 1 {
            n493 = local read "roi_current"() -> (w961:T6)
            n494 = local read "roi_sensor"() -> (w958:T6)
            n495 = Equal To 0?(x=w959) -> (x = 0?=w960:bool)
            n496 = call <userlib>:"Validate_Rect_Default.vi"("rect"=w961, "default"=w958) -> ("out"=w957:T6)
            n497 = Select(t=w957, s=w960, f=w958) -> (s? t:f=w952:T6)
            n498 = call-dynamic "CameraCheckROI.vi"("ROI_in"=w952, "CameraBase in"=w953) -> ("ROI_out"=w951:T6)  [unwired: 7 in, 2 out]
            n499 = property on="roi_capture" class="Clust (strict)"("Val(Sgnl)"=w951) -> (error out=w954:errorcluster)  [unwired: 2 in, 1 out]
            n500 = Enqueue Element(queue=w955, element=Imaging_State."Software trigger", error in (no error)=w954) -> ()  [unwired: 1 in, 3 out]
          }
          frame Default {
          }
        }
      }
      event "fit_buttons": Value Change {
        # "redraw ROIs"
        n501 = event-data() -> ("OldVal"=w968:cluster{"selection":bool, "stored":bool}, "NewVal"=w969:cluster{"selection":bool, "stored":bool})  [unwired: 1 in, 3 out]
        n502 = Cluster To Array(cluster=w968) -> (array=w970:bool[])
        n503 = Cluster To Array(cluster=w969) -> (array=w971:bool[])
        n504 = call <userlib>:"Detect_Boolean_Change.vi"("NewVal"=w971, "OldVal"=w970) -> ("ButtonId"=w966:i32)  [unwired: 2 out]
        n505 = case shown="0" w966 {
          tunnel: [_ w972] -> w963
          frame Default {
          }
          frame 0 {
            n506 = local read "roi_current"() -> (w974:T6)
            n507 = local read "fit_roi"() -> (w975:T10)
            n508 = Bundle By Name(cluster=w975, "rect"=w974) -> (w973:T10)
            n509 = property on="fit_roi" class="Clust (strict)"("Value"=w973) -> (error out=w972:errorcluster)  [unwired: 2 in, 1 out]
          }
        }
        n510 = local read "rois"() -> (w964:T7)
        n511 = property on="rois" class="Arr (strict)"(error in=w963, "Val(Sgnl)"=w964) -> (error out=w962:errorcluster)  [unwired: 1 in, 1 out]
        n512 = Enqueue Element(queue=w965, element=Imaging_State."Fit", error in (no error)=w962) -> ()  [unwired: 1 in, 3 out]
      }
      event Value Change {
        # "try to avoid infinite loop"
        n513 = event-data() -> ("CtlRef"=w986:refnum<vi>, "OldVal"=w979:T8, "NewVal"=w978:T8)  [unwired: 1 in, 2 out]
        n514 = Unbundle By Name(w978) -> ("col_scheme"=w982:u16)
        n515 = Unbundle By Name(w979) -> ("col_scheme"=w981:u16)
        n516 = Unbundle By Name(w978) -> ("val_max"=w985:sgl)
        n517 = Unbundle By Name(w979) -> ("val_max"=w984:sgl)
        n518 = Not Equal?(x=w979, y=w978) -> (x != y?=w976:bool)
        n519 = Equal?(x=w982, y=w981) -> (x = y?=w980:bool)
        n520 = Not Equal?(x=w985, y=w984) -> (x != y?=w987:bool)
        n521 = And(x=w976, y=w980) -> (x .and. y?=w977:bool)
        n522 = case shown="True" w987 {
          tunnel: w986 -> [_ w992]
          tunnel: [_ w993] -> w983
          tunnel: w978 -> [_ w990]
          frame False {
          }
          frame True {
            n523 = Bundle By Name(cluster=w990, "automax"=FALSE) -> (w991:T8)
            n524 = property class="Clust (strict)"(reference=w992, "Value"=w991) -> (error out=w993:errorcluster)  [unwired: 1 in, 1 out]
          }
        }
        n525 = case shown="True" w977 {
          tunnel: w983 -> [_ w989]
          frame False {
          }
          frame True {
            n526 = local read "frame"() -> (w988:i32)
            n527 = property on="frame" class="DigNum (strict)"(error in=w989, "Val(Sgnl)"=w988) -> ()  [unwired: 1 in, 2 out]
          }
        }
      }
      event Value Change {
        n528 = event-data() -> ("CtlRef"=w995:refnum<vi>, "NewVal"=w999:u16)  [unwired: 1 in, 3 out]
        n529 = property class="Ring (strict)"(reference=w995) -> ("Owner"=w1001:refnum<vi>)  [unwired: 1 in, 2 out]
        n530 = local read "frame"() -> (w1002:i32)
        n531 = control-ref of="raw_ctrls"() -> (w1000:refnum<vi>)
        n532 = Equal?(x=w1001, y=w1000) -> (x = y?=w998:bool)
        n533 = Greater Or Equal To 0?(x=w1002) -> (x >= 0?=w997:bool)
        n534 = Not Exclusive Or(1:w997, 2:w998) -> (0:w996:bool)
        n535 = case shown="True" w996 {
          tunnel: w999 -> [_ w1006]
          tunnel: w995 -> [_ w1003]
          frame False {
          }
          frame True {
            n536 = case shown="0" w1006 {
              tunnel: [w1010 w1018 w1019 w1020 w1022] -> w1005
              tunnel: [w1009 _ _ _ w1021] -> w1004
              tunnel: w1003 -> [w1008 _ _ _ _]
              frame Default {
                w1010 = u32 5 items=["Grayscale", "Binary", "Gradient", "Rainbow", "Temperature", "User Defined"] ("Palette:Palette Type")
                n537 = property on="Property Node" class="Ring (strict)"(reference=w1008) -> ("RingText.Text"=w1007:string)  [unwired: 1 in, 2 out]
                n538 = Concatenate Strings(w1007, ".tsv" ("string")) -> (w1011:string)
                n539 = Build Path(base path=path "Z:/Temp/rgb gradients", name or relative path=w1011) -> (appended path=w1014:path)
                n540 = call-poly <vilib>:"Read From Spreadsheet File.vi"("file path (dialog if empty)"=w1014) -> ("all rows"=w1015:dbl[][])  [unwired: 6 in, 4 out]
                n541 = for {
                  tunnel: w1015 -> [w1017] mode=indexing
                  tunnel: [w1016] -> w1009 mode=indexing
                  n542 = Array To Cluster(array=w1017) -> (cluster=w1016:T36)
                }
              }
              frame 0 {
                w1018 = u32 0 items=["Grayscale", "Binary", "Gradient", "Rainbow", "Temperature", "User Defined"] ("Palette:Palette Type")
              }
              frame 1 {
                w1019 = u32 3 items=["Grayscale", "Binary", "Gradient", "Rainbow", "Temperature", "User Defined"] ("Palette:Palette Type")
              }
              frame 2 {
                w1020 = u32 4 items=["Grayscale", "Binary", "Gradient", "Rainbow", "Temperature", "User Defined"] ("Palette:Palette Type")
              }
              frame 3 {
                n543 = property on="img_OD" class="ImageControl"() -> ("Palette Type"=w1022:u32, "User Palette"=w1021:cluster{"Red":u8, "Green":u8, "Blue":u8}[])  [unwired: 2 in, 2 out]
              }
            }
            n544 = property on="img_OD" class="ImageControl"("Palette Type"=w1005, "User Palette"=w1004) -> ()  [unwired: 2 in, 2 out]
          }
        }
      }
      event "last error.status": Value Change; "last error.status", "recent_error": Mouse Up {
        n545 = event-data() -> ("Type"=w1027:T31, "CtlRef"=w1023:refnum<vi>)  [unwired: 1 in, 2 out]
        n546 = Equal?(x=lveventtype."Mouse Up" ("Type"), y=w1027) -> (x = y?=w1025:bool)
        n547 = case shown="False" w1025 {
          tunnel: [w1029 FALSE ("recent_error")] -> w1024
          tunnel: w1023 -> [w1028 _]
          frame False {
            n548 = property on="Property Node" class="Bool (strict)"(reference=w1028) -> ("Value"=w1029:bool)  [unwired: 1 in, 2 out]
          }
          frame True {
          }
        }
        "recent_error" <- w1024
      }
      event "raw_list", "comp_list": Value Change {
        n549 = event-data() -> ("CtlRef"=w1038:refnum<vi>, "OldVal"=w1036:i32, "NewVal"=w1037:i32)  [unwired: 1 in, 2 out]
        n550 = Greater Or Equal To 0?(x=w1036) -> (x >= 0?=w1035:bool)
        n551 = Not Equal?(x=w1036, y=w1037) -> (x != y?=w1040:bool)
        n552 = Greater Or Equal To 0?(x=w1037) -> (x >= 0?=w1034:bool)
        n553 = And(x=w1040, y=w1034) -> (x .and. y?=w1039:bool)
        n554 = Exclusive Or(1:w1035, 2:w1034) -> (0:w1033:bool)
        n555 = case shown="True" w1039 {
          tunnel: w1038 -> [_ w1052]
          tunnel: w1037 -> [_ w1051]
          tunnel: w1033 -> [_ w1044]
          tunnel: [_ w1043] -> w1032
          tunnel: [w1041 w1042] -> w1031
          frame False {
            n556 = local read "frame"() -> (w1041:i32)
          }
          frame True {
            # "Set the other one to -1"
            n557 = control-ref of="raw_list"() -> (w1048:refnum<vi>)
            n558 = Equal?(x=w1048, y=w1052) -> (x = y?=w1045:bool)
            n559 = Negate(x=w1051) -> (-x=w1053:i32)
            n560 = Decrement(x=w1053) -> (x-1=w1050:i32)
            n561 = Select(t=w1051, s=w1045, f=w1050) -> (s? t:f=w1042:i32)
            n562 = control-ref of="comp_list"() -> (w1049:refnum<vi>)
            n563 = case shown="True" w1044 {
              tunnel: w1045 -> [_ w1060]
              frame False {
              }
              frame True {
                n564 = control-ref of="col_scheme"() -> (w1058:refnum<vi>)
                n565 = control-ref of="col_scheme"() -> (w1059:refnum<vi>)
                n566 = Select(t=w1059, s=w1060, f=w1058) -> (s? t:f=w1057:refnum<vi>)
                n567 = property class="Ring (strict)"(reference=w1057) -> (reference out=w1056:refnum<vi>, error out=w1055:errorcluster, "Value"=w1054:u16)  [unwired: 1 in]
                n568 = property class="Ring (strict)"(reference=w1056, error in=w1055, "Val(Sgnl)"=w1054) -> ()  [unwired: 2 out]
              }
            }
            n569 = Select(t=w1049, s=w1045, f=w1048) -> (s? t:f=w1047:refnum<vi>)
            n570 = property class="MCListbox (strict)"(reference=w1047, "Value"=-1) -> (error out=w1043:errorcluster)  [unwired: 1 in, 1 out]
          }
        }
        n571 = property on="frame" class="DigNum (strict)"(error in=w1032, "Val(Sgnl)"=w1031) -> ()  [unwired: 1 in, 2 out]
      }
      event "fit_roi": Value Change {
        w1065 = FALSE ("get")
        # "redraw ROIs"
        n572 = event-data() -> ("CtlRef"=w1063:refnum<vi>, "NewVal"=w1067:T10)  [unwired: 1 in, 3 out]
        n573 = Unbundle(w1067) -> ("get"=w1072:bool, "set"=w1071:bool, "rect"=w1068:T6)  [unwired: 1 out]
        n574 = Build Array(w1072, w1071) -> (w1070:bool[])
        n575 = Boolean Array To Number(Boolean array=w1070) -> (number=w1069:u32)
        n576 = case shown="Default" w1069 {
          tunnel: w1068 -> [w1073 _ w1075]
          tunnel: [w1073 w1074 w1075] -> w1066
          frame Default {
          }
          frame 1 {
            n577 = local read "roi_current"() -> (w1074:T6)
          }
          frame 2 {
            n578 = property on="roi_current" class="Clust (strict)"("Val(Sgnl)"=w1075) -> ()  [unwired: 2 in, 2 out]
          }
        }
        n579 = Bundle(cluster=w1067, "get"=w1065, "set"=w1065, "rect"=w1066) -> (w1064:T10)  [unwired: 1 in]
        n580 = property class="Clust (strict)"(reference=w1063, "Value"=w1064) -> (error out=w1061:errorcluster)  [unwired: 1 in, 1 out]
        n581 = local read "rois"() -> (w1062:T7)
        n582 = property on="rois" class="Arr (strict)"(error in=w1061, "Val(Sgnl)"=w1062) -> ()  [unwired: 1 in, 2 out]
      }
      event "rois": Value Change {
        n583 = event-data() -> ("CtlRef"=w1077:refnum<vi>, "NewVal"=w1079:T7)  [unwired: 1 in, 3 out]
        n584 = for {
          tunnel: w1079 -> [w1115] mode=indexing
          tunnel: [w1112] -> w1078 mode=indexing
          w1113 = FALSE ("get")
          n585 = Unbundle(w1115) -> ("get"=w1120:bool, "set"=w1119:bool, "rect"=w1116:T6)  [unwired: 1 out]
          n586 = Build Array(w1120, w1119) -> (w1118:bool[])
          n587 = Boolean Array To Number(Boolean array=w1118) -> (number=w1117:u32)
          n588 = case shown="Default" w1117 {
            tunnel: w1116 -> [w1121 _ w1123]
            tunnel: [w1121 w1122 w1123] -> w1114
            frame Default {
            }
            frame 1 {
              # "set using roi_current"
              n589 = local read "roi_current"() -> (w1122:T6)
            }
            frame 2 {
              n590 = property on="roi_current" class="Clust (strict)"("Val(Sgnl)"=w1123) -> ()  [unwired: 2 in, 2 out]
            }
          }
          n591 = Bundle(cluster=w1115, "get"=w1113, "set"=w1113, "rect"=w1114) -> (w1112:T10)  [unwired: 1 in]
        }
        n592 = property class="Arr (strict)"(reference=w1077, "Value"=w1078) -> (error out=w1076:errorcluster)  [unwired: 1 in, 1 out]
        n593 = flat-sequence {
          tunnel: w1076 -> [_]
          frame #0 {
            n594 = local read "img_OD"() -> (w1085:T4)
            n595 = call "IMAQ Clear Overlay"("Groups"=string[] ["roi"], "Image"=w1085) -> ("error out"=w1089:errorcluster, "Image Out"=w1087:T4)  [unwired: 8 in]
            n596 = call <vilib>:"Clear Errors.vi"("error in (no error)"=w1089) -> ()  [unwired: 6 in, 1 out]
            n597 = local read "roi_capture"() -> (w1090:T6)
            n598 = Build Array (concatenate)("rois", "fit_roi") -> (w1084:T7)
            n599 = Negate(x=w1090) -> (-x=w1091:T6)
            n600 = property on="x" class="DigNum (strict)"() -> ("Value"=w1081:u8)  [unwired: 2 in, 2 out]
            n601 = property on="y" class="DigNum (strict)"() -> ("Value"=w1080:u8)  [unwired: 2 in, 2 out]
            n602 = Bundle("Value"=w1081, "Value"=w1080, "Value"=w1081, "Value"=w1080) -> (w1092:T37)  [unwired: 1 in]
            n603 = for {
              tunnel: w1084 -> [w1100] mode=indexing
              shift-right: [w1097] -> w1088
              shift-left: w1087 -> [w1101]
              tunnel: w1091 -> [w1094]
              tunnel: w1092 -> [w1093]
              n604 = Unbundle By Name(w1100) -> ("color"=w1098:u32, "rect"=w1095:T6)
              n605 = Not Equal?(x=u32 16777216, y=w1098) -> (x != y?=w1096:bool)
              n606 = case shown="True" w1096 {
                tunnel: w1101 -> [w1102 w1111]
                tunnel: w1098 -> [_ w1109]
                tunnel: [w1102 w1108] -> w1097
                tunnel: w1095 -> [_ w1107]
                tunnel: w1094 -> [_ w1106]
                tunnel: w1093 -> [_ w1104]
                frame False {
                }
                frame True {
                  n607 = call <userlib>:"Apply_Rect_Offset.vi"("offset rect"=w1106, "input"=w1107) -> ("output"=w1105:T6)  [unwired: 3 in]
                  n608 = Quotient & Remainder(x=w1105, y=w1104) -> (floor(x/y)=w1103:T6)  [unwired: 1 out]
                  n609 = call "IMAQ Overlay Rectangle"("Color"=w1109, "Group"="roi", "Rectangle"=w1103, "Image"=w1111) -> ("Image Out"=w1108:T4)  [unwired: 6 in, 1 out]
                }
              }
            }
            n610 = local write "img_OD"(w1088) -> ()
          }
        }
      }
      event "frame": Value Change {
        # "redraw ROIs"
        # "Manually rescale to an I16"
        # "We've changed type, so switch color schemes"
        # "Do we actually have the frame we're supposed to show?"
        n611 = event-data() -> ("NewVal"=w1127:i32, "OldVal"=w1126:i32)  [unwired: 1 in]
        n612 = property on="image_data" class="Arr (strict)"() -> ("Value"=w1130:u16[][][])  [unwired: 2 in, 2 out]
        n613 = property on="comp_data" class="Arr (strict)"() -> ("Value"=w1131:T14)  [unwired: 2 in, 2 out]
        n614 = Less Than 0?(x=w1127) -> (x < 0?=w1150:bool)
        n615 = Less Than 0?(x=w1126) -> (x < 0?=w1128:bool)
        n616 = Equal?(x=w1127, y=w1126) -> (x = y?=w1124:bool)
        n617 = case shown="True" w1150 {
          tunnel: w1127 -> [w1160 w1167]
          tunnel: w1131 -> [_ w1170]
          tunnel: [w1158 w1165] -> w1153
          tunnel: w1130 -> [w1164 _]
          frame False {
            n618 = Array Size(array=w1164) -> (size(s)=w1163:i32[])
            n619 = Index Array(array=w1163) -> (element=w1162:i32)  [unwired: 1 in]
            n620 = Less?(x=w1160, y=w1162) -> (x < y?=w1161:bool)
            n621 = Select(t=w1160, s=w1161, f=0) -> (s? t:f=w1158:i32)
          }
          frame True {
            n622 = Negate(x=w1167) -> (-x=w1169:i32)
            n623 = Array Size(array=w1170) -> (size(s)=w1171:i32)
            n624 = Less Or Equal?(x=w1169, y=w1171) -> (x <= y?=w1168:bool)
            n625 = Select(t=w1167, s=w1168, f=0) -> (s? t:f=w1165:i32)
          }
        }
        n626 = Less Than 0?(x=w1153) -> (x < 0?=w1149:bool)
        n627 = local write "frame"(w1153) -> ()
        n628 = case shown="True" w1149 {
          tunnel: [w1176 w1179] -> w1142
          tunnel: w1153 -> [w1174 w1183]
          tunnel: [w1175 w1180] -> w1145
          tunnel: w1131 -> [_ w1178]
          tunnel: w1130 -> [w1173 _]
          tunnel: [w1172 w1177] -> w1152
          frame False {
            # "RAW DATA"
            n629 = Index Array(array=w1173, index (dim 0)=w1174) -> (element=w1176:u16[][])  [unwired: 2 in]
            n630 = control-ref of="col_scheme"() -> (w1172:refnum<vi>)
            n631 = control-ref of="raw_ctrls"() -> (w1175:refnum<vi>)
          }
          frame True {
            # "COMPUTED DATA"
            n632 = Increment(x=w1183) -> (x+1=w1182:i32)
            n633 = Negate(x=w1182) -> (-x=w1181:i32)
            n634 = Index Array(array=w1178, index=w1181) -> (element=w1184:T24)
            n635 = control-ref of="col_scheme"() -> (w1177:refnum<vi>)
            n636 = control-ref of="comp_ctrls"() -> (w1180:refnum<vi>)
            n637 = Unbundle By Name(w1184) -> ("data"=w1179:sgl[][])
          }
        }
        n638 = Exclusive Or(1:w1128, 2:w1149) -> (0:w1151:bool)
        n639 = Or(x=w1124, y=w1151) -> (x .or. y?=w1125:bool)
        n640 = case shown="True" w1125 {
          tunnel: w1152 -> [_ w1157]
          frame False {
          }
          frame True {
            n641 = property class="Ring (strict)"(reference=w1157) -> (reference out=w1156:refnum<vi>, error out=w1154:errorcluster, "Value"=w1155:u16)  [unwired: 1 in]
            n642 = property class="Ring (strict)"(reference=w1156, error in=w1154, "Val(Sgnl)"=w1155) -> ()  [unwired: 2 out]
          }
        }
        n643 = property class="Clust (strict)"(reference=w1145) -> (reference out=w1143:refnum<vi>, "Value"=w1146:T8)  [unwired: 1 in, 1 out]
        n644 = Unbundle By Name(w1146) -> ("automax"=w1148:bool, "val_max"=w1144:sgl, "val_min"=w1147:sgl)
        n645 = Subtract(x=w1142, y=w1147) -> (x-y=w1139:sgl[][])
        n646 = case shown="True" w1148 {
          tunnel: [w1185 w1188] -> w1135
          tunnel: w1142 -> [_ w1190]
          tunnel: w1143 -> [_ w1189]
          tunnel: w1144 -> [w1185 _]
          tunnel: w1146 -> [_ w1186]
          frame False {
          }
          frame True {
            # "Recompute maximum value"
            n647 = Array Max & Min(array=w1190) -> (max value=w1188:sgl)  [unwired: 3 out]
            n648 = Bundle By Name(cluster=w1186, "val_max"=w1188) -> (w1187:T8)
            n649 = property class="Clust (strict)"(reference=w1189, "Value"=w1187) -> ()  [unwired: 1 in, 2 out]
          }
        }
        n650 = Subtract(x=w1135, y=w1147) -> (x-y=w1136:sgl)
        n651 = Divide(x=sgl 32767.0, y=w1136) -> (x/y=w1138:sgl)
        n652 = Multiply(x=w1139, y=w1138) -> (x*y=w1140:sgl[][])
        n653 = local read "img_OD"() -> (w1132:T4)
        n654 = To Word Integer(number=w1140) -> (16bit integer=w1129:i16[][])
        n655 = local read "rois"() -> (w1134:T7)
        n656 = call "IMAQ ArrayToImage"("Image Pixels (I16)"=w1129, "Image"=w1132) -> ("error out"=w1133:errorcluster, "Image Out"=w1141:T4)  [unwired: 8 in]
        n657 = local write "img_OD"(w1141) -> ()
        n658 = property on="rois" class="Arr (strict)"(error in=w1133, "Val(Sgnl)"=w1134) -> ()  [unwired: 1 in, 2 out]
      }
    }
  }
  n659 = while {
    tunnel: w35 -> [w1199]
    tunnel: w24 -> [w1193]
    tunnel: w36 -> [w1192]
    tunnel: w1 -> [w1191]
    stop <- FALSE stop-if-true
    # "Wait for TCP"
    # "Run forever"
    n660 = TCP Wait On Listener(11:w1199) -> (0:w1196:errorcluster, 1:w1197:u16, 2:w1198:string, 4:w1194:refnum<k5>)  [unwired: 3 in, 1 out]
    n661 = Format Into String(format string=":%d", initial string=w1198, w1197) -> (resulting string=w1200:string)  [unwired: 1 in, 1 out]
    n662 = case shown="No Error" w1196 {
      selector: w1196 -> [_ w1328]
      tunnel: w1194 -> [w1227 _]
      tunnel: w1200 -> [w1222 _]
      tunnel: w1192 -> [w1209 _]
      tunnel: w1193 -> [w1208 _]
      tunnel: w1191 -> [w1204 _]
      frame No Error {
        # "Receive data"
        n663 = TCP Read(connection ID=w1227, bytes to read=1024, 7:T38."CRLF" ("mode (standard)"), 9:500 ("timeout ms (25000)")) -> (connection ID out=w1220:refnum<k5>, data out=w1224:string)  [unwired: 1 in, 1 out]
        n664 = Dequeue Element(queue=w1204, timeout in ms (-1)=100) -> (queue out=w1203:refnum<queue>, element=w1202:errorcluster)  [unwired: 1 in, 2 out]
        n665 = call <vilib>:"Trim Whitespace.vi"("string"=w1224) -> ("trimmed string"=w1223:string)  [unwired: 1 in]
        n666 = case shown="Default" w1223 {
          selector: w1223 -> [w1273 _ _ _]
          tunnel: w1222 -> [w1272 _ _ _]
          tunnel: [_ "done\r\n" ("data in") "hello\r\n" ("data in") _] -> w1212
          tunnel: w1209 -> [w1269 w1318 w1321 w1326]
          tunnel: w1208 -> [w1268 w1317 _ _]
          tunnel: [w1267 w1314 w1319 w1324] -> w1210
          tunnel: [w1266 w1315 w1321 w1323] -> w1206
          tunnel: w1203 -> [w1262 w1309 _ _]
          tunnel: w1202 -> [w1261 w1308 w1319 w1322]
          frame Default {
            n667 = String To Path(string=w1273) -> (path=w1265:path)
            n668 = Get Date/Time In Seconds() -> (seconds since 1Jan1904=w1271:timestamp)
            n669 = call <vilib>:"H5Fis_hdf.vi"("path in"=w1265) -> ("error out"=w1263:errorcluster, "valid?"=w1264:bool)  [unwired: 7 in, 2 out]
            n670 = Format Into String(format string="Received \"%s\" from %s at %T", w1273, w1272, w1271) -> (resulting string=w1270:string)  [unwired: 2 in, 1 out]
            n671 = case shown="False" w1264 {
              tunnel: w1265 -> [w1279 w1294]
              tunnel: w1269 -> [w1276 w1285]
              tunnel: [w1281 w1292] -> w1267
              tunnel: w1268 -> [_ w1295]
              tunnel: [w1276 w1291] -> w1266
              tunnel: w1263 -> [_ _]
              tunnel: w1262 -> [_ w1283]
              tunnel: w1261 -> [w1275 w1282]
              frame False {
                n672 = Format Into String(format string="Received file \"%s\" not a valid HDF ", w1279) -> (resulting string=w1278:string)  [unwired: 2 in, 1 out]
                n673 = call <vilib>:"Error Cluster From Error Code.vi"("error in (no error)"=w1275, "error message (\"\")"=w1278, "error code (0)"=6042 ("t")) -> ("error out"=w1281:errorcluster)  [unwired: 6 in]
              }
              frame True {
                n674 = call-dynamic "CameraAbort.vi"("CameraBase in"=w1295) -> ("error out"=w1290:errorcluster)  [unwired: 9 in, 1 out]
                n675 = Dequeue Element(queue=w1283, timeout in ms (-1)=100, error in (no error)=w1290) -> (element=w1287:errorcluster, error out=w1288:errorcluster)  [unwired: 2 out]
                n676 = Flush Queue(queue=w1285) -> (queue out=w1293:refnum<queue>, error out=w1286:errorcluster)  [unwired: 1 in, 1 out]
                n677 = Merge Errors(w1282, w1287, w1288, w1286) -> (w1284:errorcluster)
                n678 = case shown="Error" w1284 {
                  selector: w1284 -> [_ w1306]
                  tunnel: w1294 -> [w1305 _]
                  tunnel: w1293 -> [w1304 w1307]
                  tunnel: [w1299 w1306] -> w1292
                  tunnel: [w1298 w1307] -> w1291
                  frame No Error {
                    n679 = Strip Path(path=w1305) -> (stripped path=w1297:path, name=w1296:string)
                    n680 = Enqueue Element(queue=w1304, element=Imaging_State."Read File") -> (queue out=w1302:refnum<queue>, error out=w1300:errorcluster)  [unwired: 2 in, 1 out]
                    n681 = local write "working dir"(w1297) -> ()
                    n682 = local write "current file"(w1296) -> ()
                    n683 = Enqueue Element(queue=w1302, element=Imaging_State."Acquire", error in (no error)=w1300) -> (queue out=w1298:refnum<queue>, error out=w1299:errorcluster)  [unwired: 1 in, 1 out]
                  }
                  frame Error {
                  }
                }
              }
            }
            n684 = call <userlib>:"BasicLogger.vi"("text"=w1270) -> ()  [unwired: 6 in, 2 out]
          }
          frame "abort" {
            # "BLACS signals abort"
            # "Kill the queue"
            # "Abort the camera"
            n685 = call-dynamic "CameraAbort.vi"("CameraBase in"=w1317) -> ("error out"=w1310:errorcluster)  [unwired: 9 in, 1 out]
            n686 = Dequeue Element(queue=w1309, timeout in ms (-1)=100, error in (no error)=w1310) -> (element=w1312:errorcluster, error out=w1313:errorcluster)  [unwired: 2 out]
            n687 = Merge Errors(w1308, w1312, w1313) -> (w1314:errorcluster)
            n688 = Flush Queue(queue=w1318) -> (queue out=w1315:refnum<queue>)  [unwired: 1 in, 2 out]
          }
          frame "hello" {
          }
          frame "done" {
            n689 = Enqueue Element(queue=w1326, element=Imaging_State."Save File", error in (no error)=w1322) -> (queue out=w1323:refnum<queue>, error out=w1324:errorcluster)  [unwired: 1 in, 1 out]
            n690 = call <userlib>:"BasicLogger.vi"("text"="Received \"done\" command") -> ()  [unwired: 6 in, 2 out]
          }
        }
        n691 = case shown="Default" w1212 {
          selector: w1212 -> [w1241 _]
          tunnel: w1220 -> [w1242 w1258]
          tunnel: [w1242 w1255] -> w1216
          tunnel: [w1241 "done\r\n"] -> w1215
          tunnel: [w1240 w1244] -> w1211
          tunnel: w1210 -> [w1240 w1249]
          tunnel: w1203 -> [_ w1243]
          frame Default {
          }
          frame "" {
            # "Send acknowledge response"
            n692 = Dequeue Element(queue=w1243, timeout in ms (-1)=20000, error in (no error)=w1249) -> (element=w1246:errorcluster, timed out?=w1248:bool, error out=w1247:errorcluster)  [unwired: 1 out]
            n693 = TCP Write(connection ID=w1258, data in="ok\r\n", 9:500 ("timeout ms (25000)")) -> (connection ID out=w1255:refnum<k5>, error out=w1260:errorcluster)  [unwired: 1 in, 1 out]
            n694 = Merge Errors(w1247, w1246) -> (w1245:errorcluster)
            n695 = call <vilib>:"Clear Errors.vi"("error in (no error)"=w1260) -> ()  [unwired: 6 in, 1 out]
            n696 = Select(t=6040, s=w1248, f=0 ("error code (0)")) -> (s? t:f=w1252:i32)
            n697 = call <vilib>:"Error Cluster From Error Code.vi"("error in (no error)"=w1245, "error message (\"\")"="Imaging system timed out" ("error message (\"\")"), "error code (0)"=w1252) -> ("error out"=w1244:errorcluster)  [unwired: 6 in]
          }
        }
        n698 = case shown="Error" w1211 {
          selector: w1211 -> [w1234 _]
          tunnel: [w1232 w1239] -> w1219
          tunnel: w1215 -> [_ w1239]
          tunnel: w1206 -> [w1230 _]
          tunnel: [w1229 _] -> _
          tunnel: [_ FALSE] -> w1207
          tunnel: w1203 -> [w1228 _]
          frame Error {
            w1233 = T16 0 items=["no dialog", "OK message", "continue or stop message", "OK message + warnings", "continue/stop + warnings"] ("type of dialog (OK msg:1)")
            # "kill any commands in the queue"
            # "Check if any errors occurred\nIf they did, BLACS will want to know"
            n699 = Flush Queue(queue=w1230) -> ()  [unwired: 1 in, 3 out]
            n700 = Flush Queue(queue=w1228) -> ()  [unwired: 1 in, 3 out]
            n701 = call <vilib>:"Simple Error Handler.vi"("type of dialog (OK msg:1)"=w1233, "error in (no error)"=w1234) -> ("error out"=w1231:errorcluster, "message"=w1235:string)  [unwired: 3 in, 3 out]
            n702 = Concatenate Strings("ERROR: " ("string"), w1235) -> (w1232:string)
            n703 = call <userlib>:"BasicErrorLogger.vi"("error in"=w1231) -> ("error out"=w1229:errorcluster)  [unwired: 1 in, 1 out]
          }
          frame No Error {
            n704 = Wait (ms)(milliseconds to wait=u32 100) -> ()  [unwired: 1 out]
          }
        }
        n705 = local write "remote"(w1207) -> ()
        n706 = TCP Write(connection ID=w1216, data in=w1219, 9:500 ("timeout ms (25000)")) -> (connection ID out=w1214:refnum<k5>, error out=w1217:errorcluster)  [unwired: 1 in, 1 out]
        n707 = TCP Close Connection(connection ID=w1214, error in (no error)=w1217) -> (error out=w1221:errorcluster)  [unwired: 1 in, 1 out]
        n708 = call <vilib>:"Clear Errors.vi"("error in (no error)"=w1221) -> ()  [unwired: 6 in, 1 out]
      }
      frame Error {
        n709 = call <userlib>:"BasicErrorLogger.vi"("error in"=w1328) -> ()  [unwired: 1 in, 2 out]
      }
    }
  }
  n710 = Stop(stop? (T)=w38) -> ()
  "acquiring" <- w26
